vi "main_b.vi"(8 "error in (no error)":errorcluster, 10 "stages":refnum<class "_stage.lvclass">[](array[class]), 11 "_camera":refnum<class "_camera.lvclass">) -> ()   [LabVIEW 2019]
uses:
  _camera/_camera.lvlibp/_cameraClass/_camera.lvclass
  _stage/_stage.lvlibp/_stageClass/_stage.lvclass
  data_algorithm.ctl
  state.ctl
  data_process.ctl
  _data/_data.lvlibp/_dataClass/_data.lvclass
  <vilib>/Analysis/baseanly.llb/Mean (DBL).vi
  972fad81-3ff3-4c5b-b5d6-c93ea4aec52b.vi
  951adbdd-488d-47b0-b06c-8d69e9ccb4aa.vi
  2b97118a-447f-4295-80f1-8ed8751fa7ac.vi
  <vilib>/Utility/config.llb/Read Key (Path).vi
  <vilib>/Utility/config.llb/Read Key (String).vi
  _camera/_camera.lvlibp/_cameraClass/Write stage positions readback.vi
  _camera/_camera.lvlibp/_cameraClass/Write config file path.vi
  _camera/_camera.lvlibp/_cameraClass/Read camera name and version.vi
  _camera/_camera.lvlibp/_cameraClass/Write background.vi
  _camera/_camera.lvlibp/_cameraClass/Read wavelength.vi
  <vilib>/gmath/NumericalOptimization/Nonlinear Curve Fit LM formula string.vi
  _camera/_camera.lvlibp/_cameraClass/Write wavelength.vi
  _camera/_camera.lvlibp/_cameraClass/Read stage positions.vi
  _camera/_camera.lvlibp/_cameraClass/Write stage positions.vi
  <vilib>/Utility/file.llb/Read Delimited Spreadsheet (DBL).vi
  <vilib>/Utility/config.llb/Read Key (Double).vi
  <vilib>/Analysis/NI_AALBase.lvlib
  <vilib>/Utility/config.llb/NI_LVConfig.lvlib
  <vilib>/gmath/NI_Gmath.lvlib
  378a35e6-17c3-42fc-973f-4dbb75f37032.vi
  <vilib>/Utility/LVLibp/NI_PackedLibraryUtility.lvlib
panel:
  out "concatenated string":string
  out "t/out":bool
  in  "Tab Control 2":enum32{"Page 1", "Page 2"}(tab)
  out "number (0 to 1) 3":dbl
  in  "calibrate wavelength":bool caption="calibrate_wl"
  out "Boolean 3":bool
  out "number (0 to 1) 2":dbl
  out "number (0 to 1)":dbl
  out "size of dependent time scan":i32
  out "single acq. time":u32
  out "data proc. time":u32=150 caption="usec"
  in  "which plot":u16(ring)=2 items=["pumped", "unpumped", "reference", "difference"]
  in  "Algorithm":T1=3 items=["<(S*-S)/S>/ln(10)", "<S*/S>-1", "<S*/PD*>/<S/PD>", "<S*/Sref*>/<S/Sref>", "<S*/Sref*/PD*>/<S/Sref>", "<S*/Sref*>/<S/Sref>_alt"]
  in  "show reference spectrum?":bool
  in  "remove cursor":bool
  in  "add cursor":bool
  out "Array":i32[](array[numeric])
  out "x = y?":bool
  in  "reversed?":bool[](array[boolean])=[TRUE]
  in  "Experimenter":string="who are you?"
  in  "Title":string="A clever title"
  in  "Experimental parameters":string="sample:\nsolvent:\ncuvette:\noptical density:\nexcitation wavelength:\nexcitation power:\nexcitation spot size:\nexcitation fluence: \nprobe spot size:\ncomment:"
  out "current scan":i32
  in  "N scans":u16=5
  in  "sample":string="testSample"
  in  "Experiment":string="testExp"
  in  "center cursor":bool
  in  "save flag":bool
  in  "save type":bool[](array[boolean])=[FALSE, FALSE, FALSE, FALSE]
  in  "data folder":path=path "Z:/11 Setups/04 NOPA TA/01 Data"
  out "progress":dbl(slide)=21.0 scale=0.0..100.0
  out "scan progress":u8(slide)=16 scale=0.0..100.0
  out "Cursor position (wl)":dbl[](array[numeric]) format="%#.2g"
  out "Cursor position (idx)":dbl[](array[numeric])
  in  "ampl":cluster{dbl, dbl}(slide)={-0.2917505030181087, 6.9678068410462775} scale=-1.0..10.0
  in  "diff":dbl(slide)=26.28128772635815 scale=0.05..50.0
  out "main graph":cluster{"wavelength":dbl[], "ref mean":dbl[]}[](graph)
  out "Tab Control":T2(tab)
  out "Intensity Chart":dbl[][](graph)
  out "Intensity Graph":dbl[][](graph)
  out "Waveform Chart":T3(graph)
  out "std graph":cluster{"wavelength":dbl[], "ref std":dbl[]}[](graph)
  out "std":dbl
  out "std":dbl
  out "skipped":bool[](array[boolean])
  out "chopper out":bool[][](array[boolean])
  out "synchronization error":bool
  out "mean":dbl
  out "mean":dbl
  out "PD hist":T4(graph)
  out "PD":cluster{i32[], dbl[]}[](graph)
  in  "ts_plot_lin-log":bool caption="timestep_plot_linlog"
  out "base path":path
  out "stage config":path
  out "camera config":path
  out "Application Directory":path
  out "appended path":path
  out "Stage objects":refnum<class "_stage.lvclass">[](array[class])
  out "timesteps loaded from file":dbl[][](array[numeric])
  out "size of dependent time scan 2":i32
  out "Waveform Graph":dbl[](graph)
  in  "trig2 level":dbl(slide)=783.9195979899498 scale=0.0..2000.0
  out "Tank 2":dbl(slide) scale=0.0..2000.0
  out "Tank 2 + std":dbl(slide) scale=0.0..2000.0
  out "Tank 2 - std":dbl(slide) scale=0.0..2000.0
  in  "trig1 level":dbl(slide)=783.9195979899498 scale=0.0..2000.0
  out "Tank 1":dbl(slide)=552.7638190954774 scale=0.0..2000.0
  out "Tank 1 - std":dbl(slide) scale=0.0..2000.0
  out "Tank 1 + std":dbl(slide) scale=0.0..2000.0
  in  "baseline offset (ref.)":dbl
  in  "baseline offset (signal)":dbl
  in  "history length":i32=20
  in  "Scale.Range:Maximum":dbl(slide)=43.976036093027226 caption="diff scale range" scale=1.0..1000.0
  in  "camera max scale":u16(ring) items=["16-bit", "14-bit", "12-bit"]
  in  "save raw data":bool caption="saw raw data"
  in  "is measurement TA?":bool=TRUE
  out "Boolean 2":bool
  out "element 2":dbl
  out "element 3":dbl
  out "PDs mean":dbl[](array[numeric])
  out "PDs std":dbl[](array[numeric])
  out "dynamic offset":dbl[](array[numeric])
  in  "use dynamic offset?":bool
  in  "save wl calibration to .ini":bool caption="calibrate_wl"
  in  "index":u16
  out "wavelength fit":cluster{i32[], dbl[]}[](graph)
  out "wavelength (fitted)":dbl[](array[numeric]) format="%#.0f"
  in  "wavelength \n(calibration value)":dbl[](array[numeric]) caption="wavelength (calibration value)"
  in  "pixel/index":u16[](array[numeric])
  in  "mirror?":bool
  in  "initial parameters":dbl[](array[numeric])=[150.0, 200000.0, 1200.0]
  out "best fit parameters":dbl[](array[numeric])
  in  "time delay file":path=path "D:/github/TransientAbsorptionDAQ.lv/stepfiles/01_coarseSteps_-1000_1000fs.txt"
  in  "scan":bool
  in  "bottom panel":u16(ring)=2 items=["x/y", "y/x", "traces", "std", "debug", "debug 2", "parameters", "wavelength"]
  in  "parity?":enum32{"Item 0", "Item 1"}(radio)
  out "Camera initialised?":bool[](array[boolean])
  out "Char":i16
  in  "view error anal":bool
  in  "view full data":bool
  in  "get bg":bool
  in  "cont acq":bool
  in  "move stage":enum32{"Item 0", "Item 1"}(radio)
  out "timed out?":bool
  out "Boolean":bool
  out "Stage(s) initialized":bool[](array[boolean])
  in  "set as t0":bool[](array[boolean])
  in  "home stages":bool[](array[boolean])
  out "stage name(s)":i32[](listbox)
  in  "t0 position(s)":dbl[](array[numeric]) caption="t0 (s)" format="%07.0f"
  out "stage position(s) readback":dbl[](array[numeric]) caption="readback (fs)" format="%09.2f"
  in  "stage position(s)":dbl[](array[numeric]) caption="set (fs)" format="%07.0f"
  out "camera name, version":string
  in  "get_single_acq":bool caption="get single"
  out "vi running?":bool=TRUE
  out "is moving?":bool[](array[boolean]) caption="mov?"
  # "scan"
  # "out of"
  # "just temp ..."
  # "timing"
  # "usec"
  # "transient"
  # "pumped mean"
  # "unpumped mean"
  # "reference mean"
  # "Hartmann dispersion formula:"
  # "d(\\lambda) = a1 + a2 / (pix - a3)"
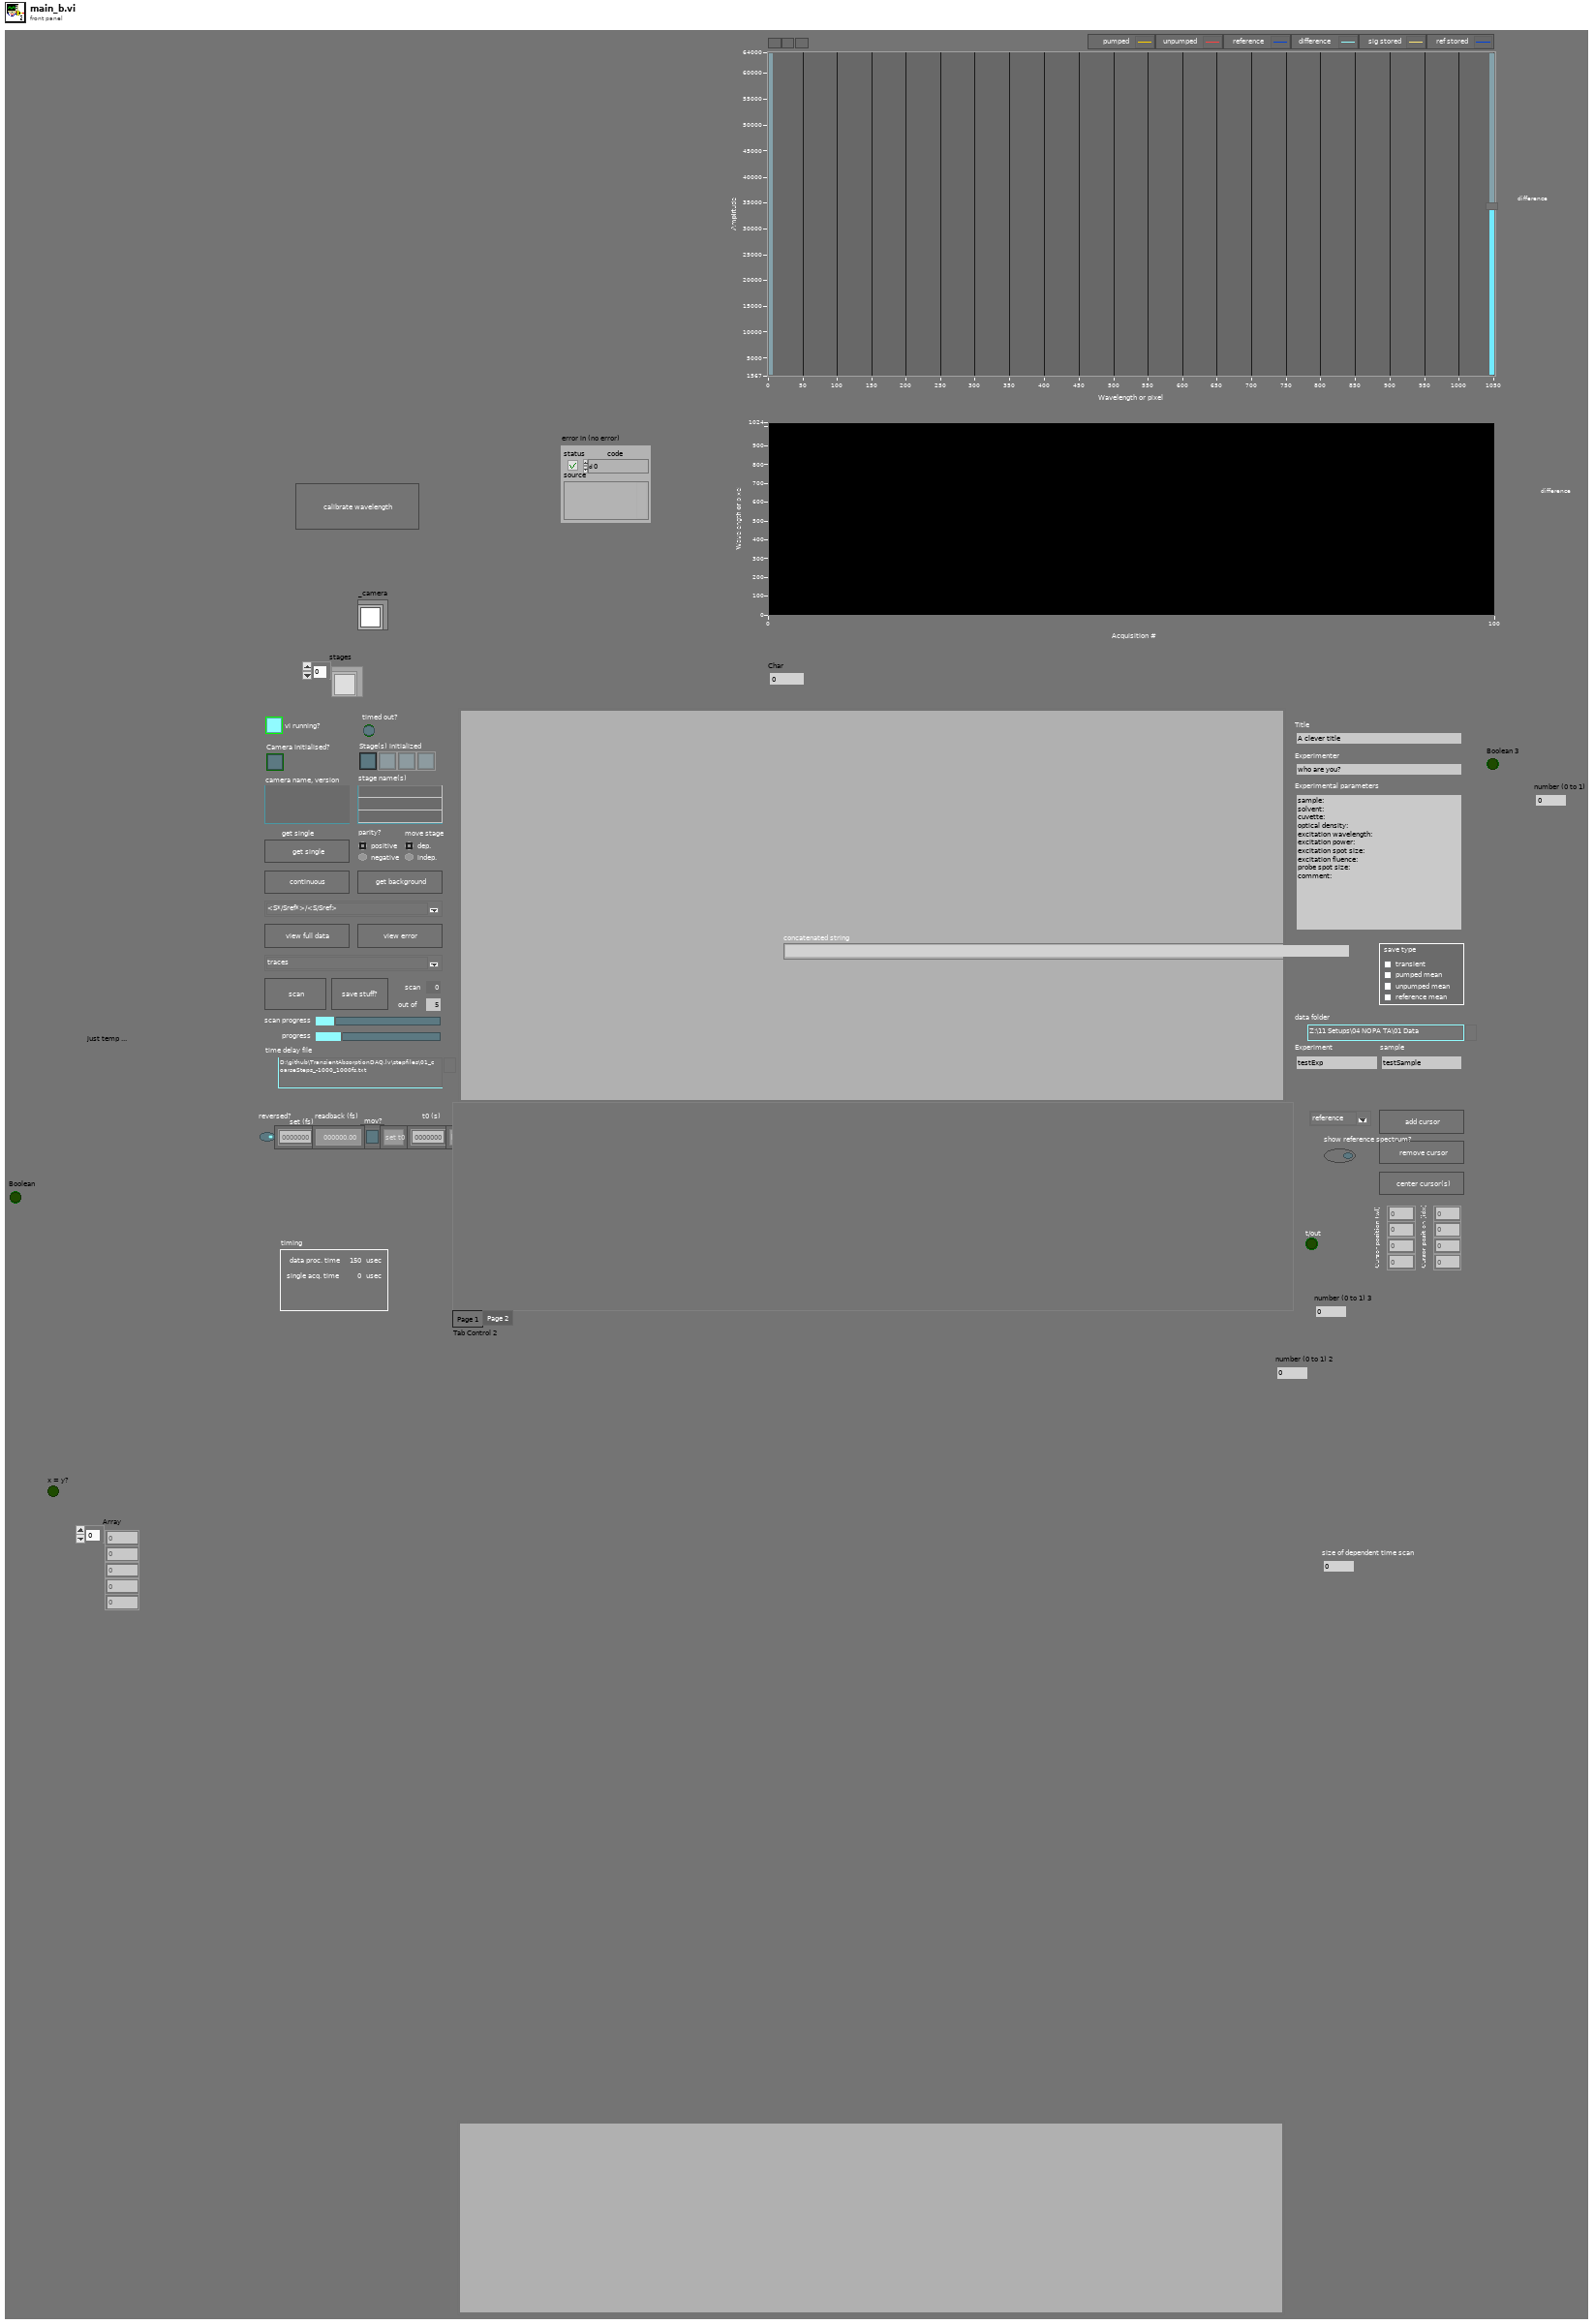
[diagram p1: front panel]
types:
  T1 = typedef "data_algorithm.ctl" = u16
  T2 = enum32{"x/y", "y/x", "traces", "std", "debug", "debug 2", "parameters", "wavelength"}
  T3 = cluster{"[0]":dbl, "[1]":dbl, "[2]":dbl, "[3]":dbl, "[4]":dbl, "[5]":dbl, "[6]":dbl, "[7]":dbl, "[8]":dbl}
  T4 = cluster{"Histogram: h(x)":i32[], "X Values":dbl[]}[]
  T5 = enum32{"invalid app kind", "Development System", "Run Time System", "Student Edition", "Embedded LabVIEW", "Evaluation", "Custom"}
  T6 = typedef "data_process.ctl" = enum16{"timeout", "init", "reset", "process", "plot", "save", "exit"}
  T7 = cluster{"type":string, "raw data":dbl[][][], "wavelength":dbl[], "trigger":bool[][], "stage position (set) [fs]":dbl[], "stage position (readback) [fs]":dbl[], "scn_step_pos (set)":dbl[], "scn_step_time_dly (set) [fs]":dbl[][], "scn_step":i32, "scn_iter":i32, "command":T6, "save flag":bool, "save path":path, "save type":bool[], "raw PDs":dbl[][]}
  T8 = typedef "state.ctl" = enum16{"timeout", "hw_init", "sw_init", "cam_single_acq", "cam_get_bg", "cam_rst_bg", "cam_cnt_acq", "cam_set_wl", "stg_set_pos", "stg_home", "scn_load_step_file", "scn_init", "scn_next_step", "scn_next_iter", "dat_update_save_flag", "dat_update_save_type", "dat_save_raw", "dat_send_to_process", "aux_save_wl_to_ini", "aux_center_cursor", "stop"}
  T9 = cluster{"acq num":u32[], "curr acq":i32, "signal":dbl[], "signal (accum.)":dbl[][], "pumped mean":dbl[], "unpumped mean":dbl[], "reference mean":dbl[], "pumped std":dbl[], "unpumped std":dbl[], "reference std":dbl[], "pumped stored":dbl[], "reference stored":dbl[], "signal std":dbl[]}
  T10 = typedef "NI_LVConfig.lvlib/Config Data RefNum.ctl" = refnum<k1>
  T11 = typedef "LVRangeTypeDef.ctl" = cluster{"Minimum":dbl, "Maximum":dbl, "Increment":dbl, "Minor Increment":dbl, "Start":dbl}
  T12 = typedef "LVCursorListTypeDef.ctl" = cluster{"Name":string, "Color":u32, "Style":u8, "Point Style":u8, "Name Visible":bool, "Allow Drag":bool, "Cursor Mode":u32, "Plot":i32, "Index":i32, "Position":cluster{"X":dbl, "Y":dbl}, "X Scale":u32, "Y Scale":u32, "Watch Plots":i32[], "Watch All Plots":bool, "Plot Area":i32, "Label Offset":cluster{"X":dbl, "Y":dbl}}[]
  T13 = cluster{"Name":string, "Color":u32, "Style":u8, "Point Style":u8, "Name Visible":bool, "Allow Drag":bool, "Cursor Mode":u32, "Plot":i32, "Index":i32, "Position":cluster{"X":dbl, "Y":dbl}, "X Scale":u32, "Y Scale":u32, "Watch Plots":i32[], "Watch All Plots":bool, "Plot Area":i32, "Label Offset":cluster{"X":dbl, "Y":dbl}}
  T14 = cluster{"wavelength":dbl[], "unpumped mean":dbl[]}
  T15 = cluster{"wavelength":dbl[], "reference mean":dbl[]}
  T16 = cluster{"wavelength":dbl[], "reference stored":dbl[]}
  T17 = cluster{"wavelength":dbl[], "pumped stored":dbl[]}
  T18 = cluster{"Histogram: h(x)":i32[], "X Values":dbl[]}
  T19 = cluster{"wavelength":dbl[], "reference stored":dbl[]}[]
  T20 = cluster{"wavelength":dbl[], "unpumped std":dbl[]}
  T21 = cluster{"wavelength":dbl[], "reference std":dbl[]}
  T22 = cluster{"wavelength":dbl[], "reference std":dbl[]}[]
  T23 = cluster{"model":string, "Parameters":string[], "x":string}
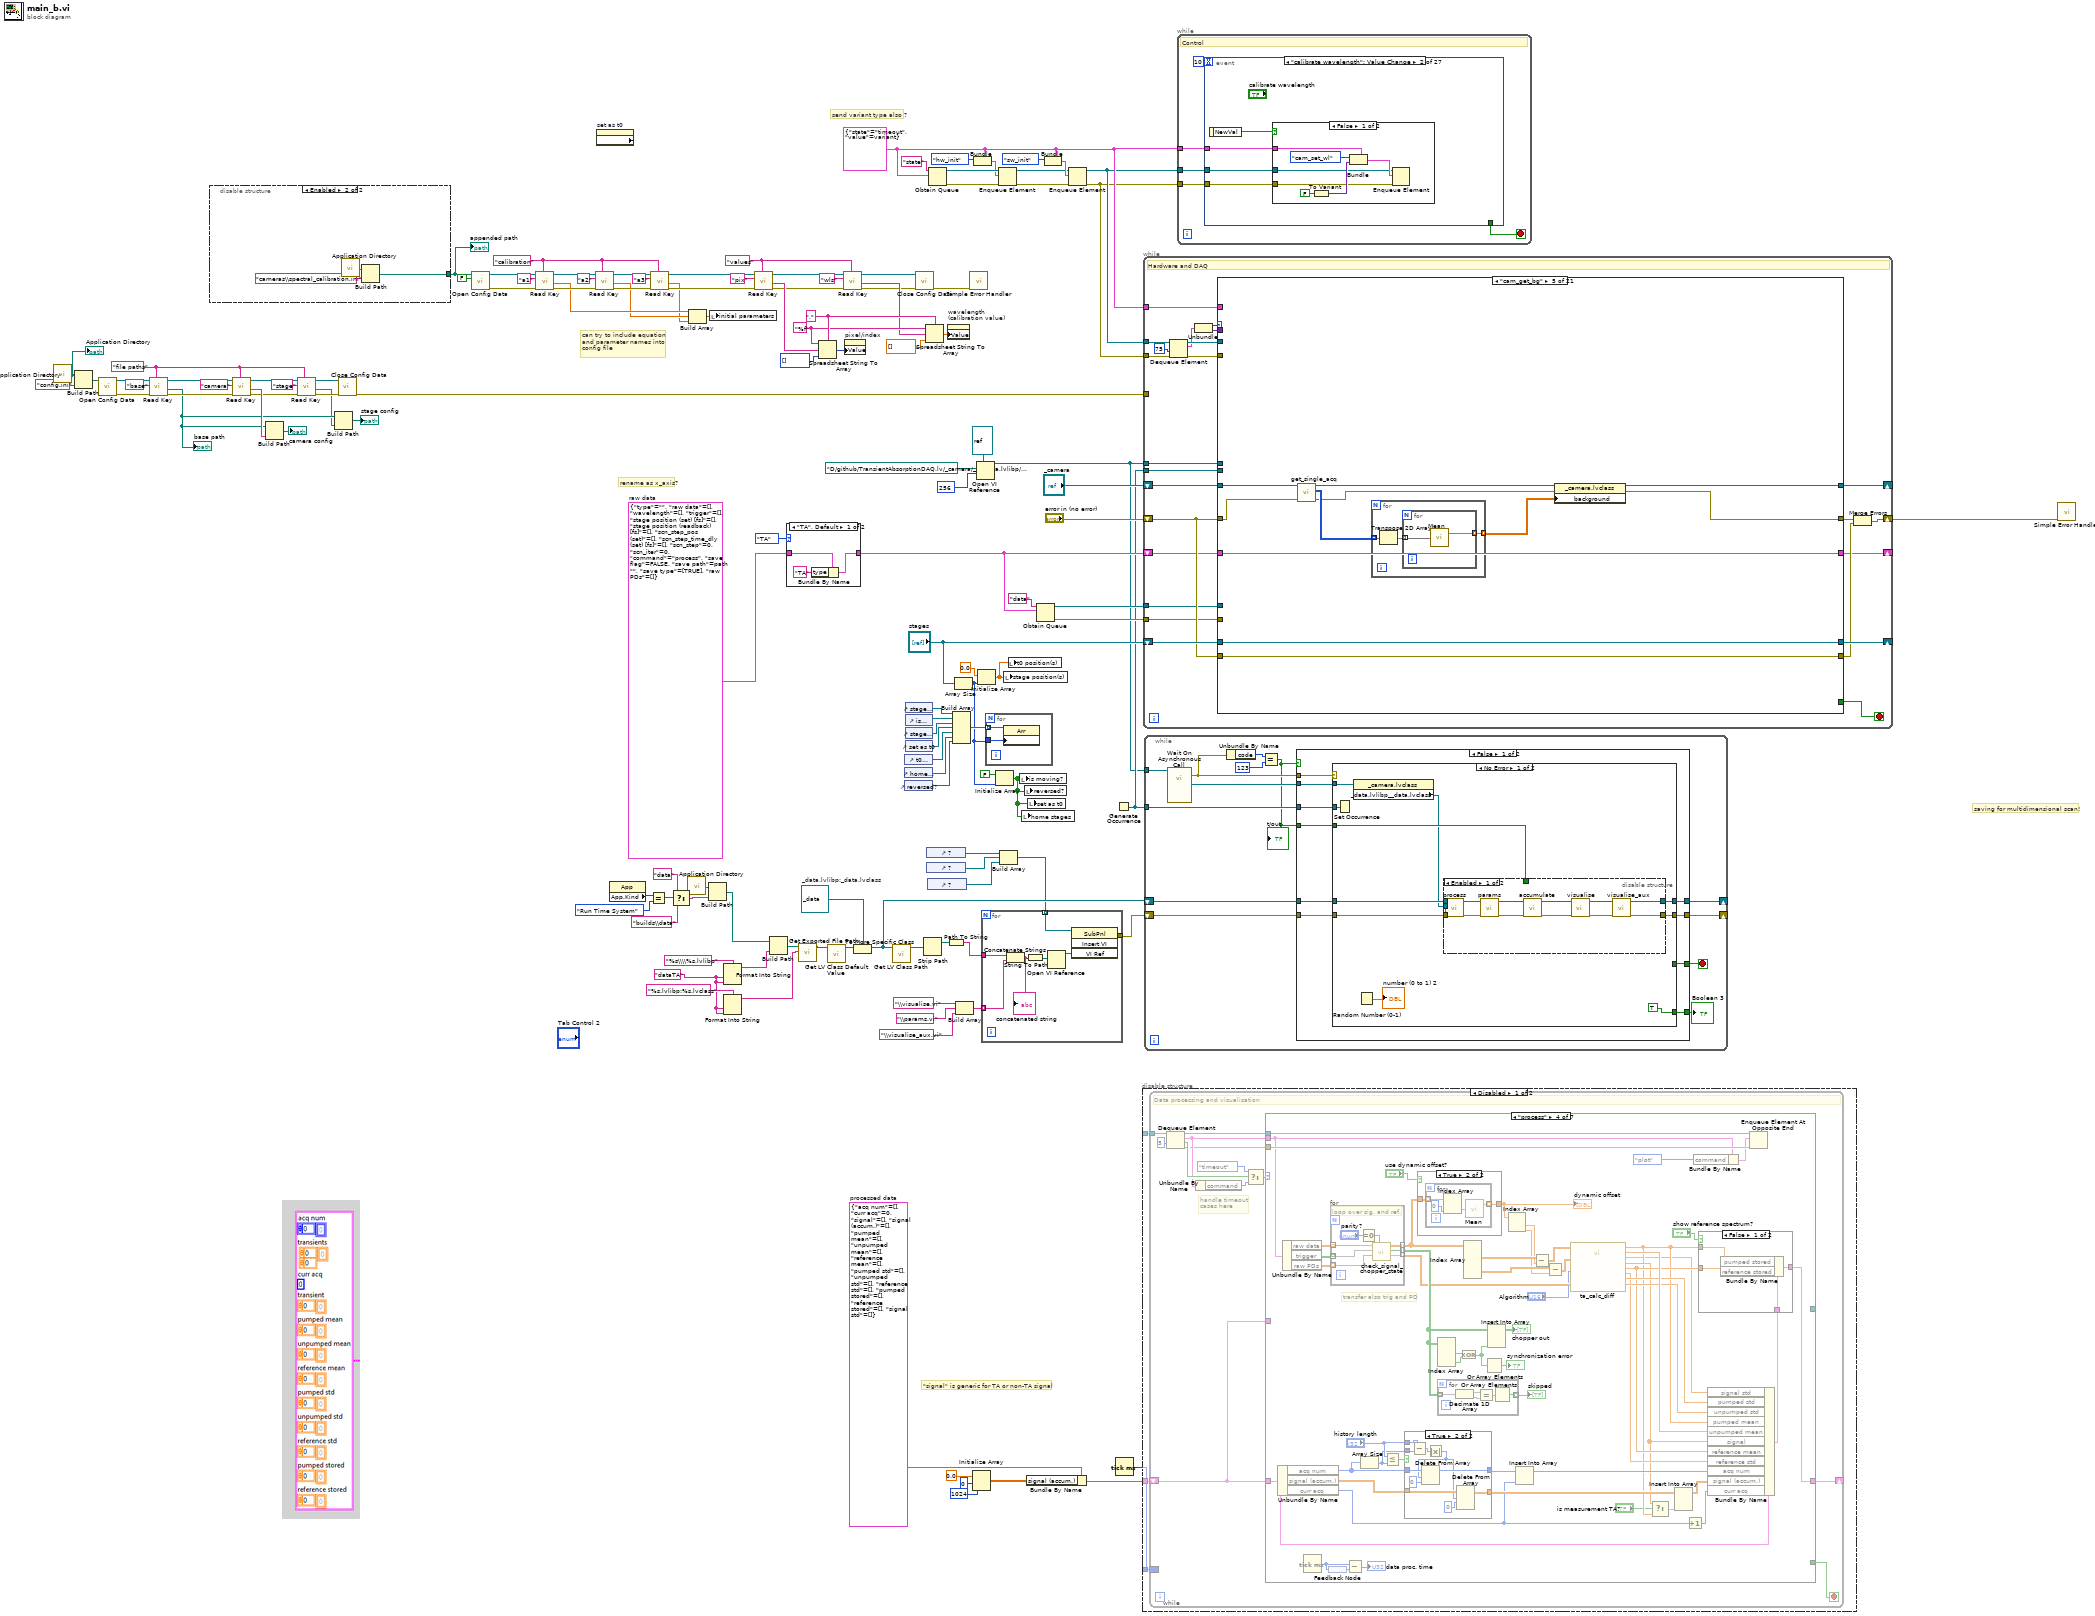
[diagram p0: block diagram]
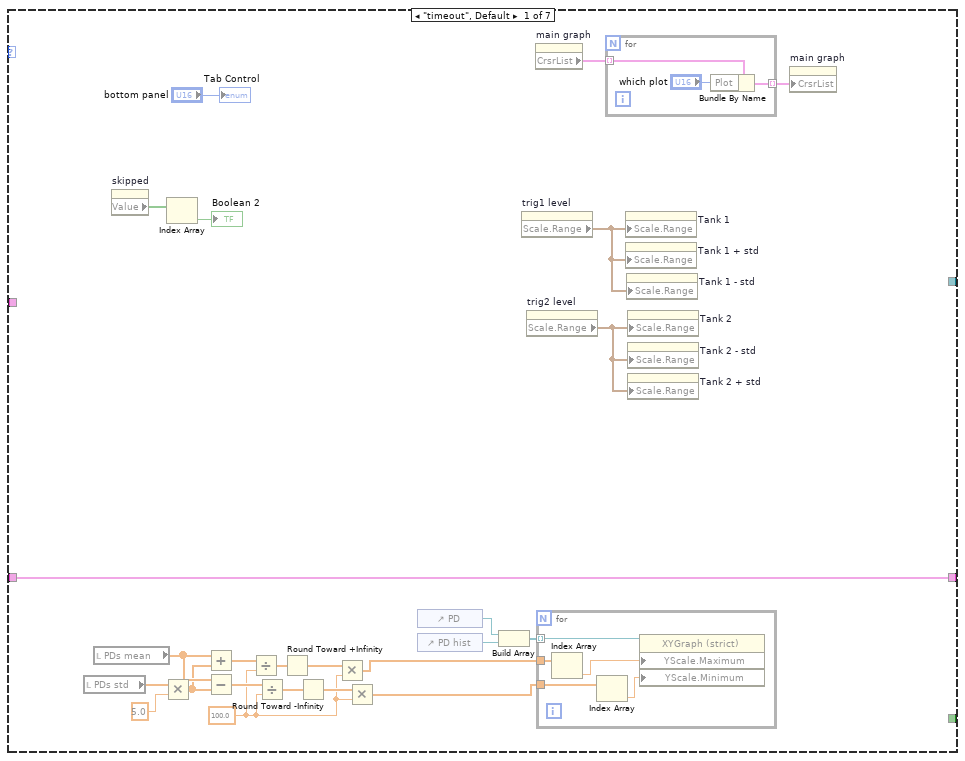
[diagram p2: hidden frame]
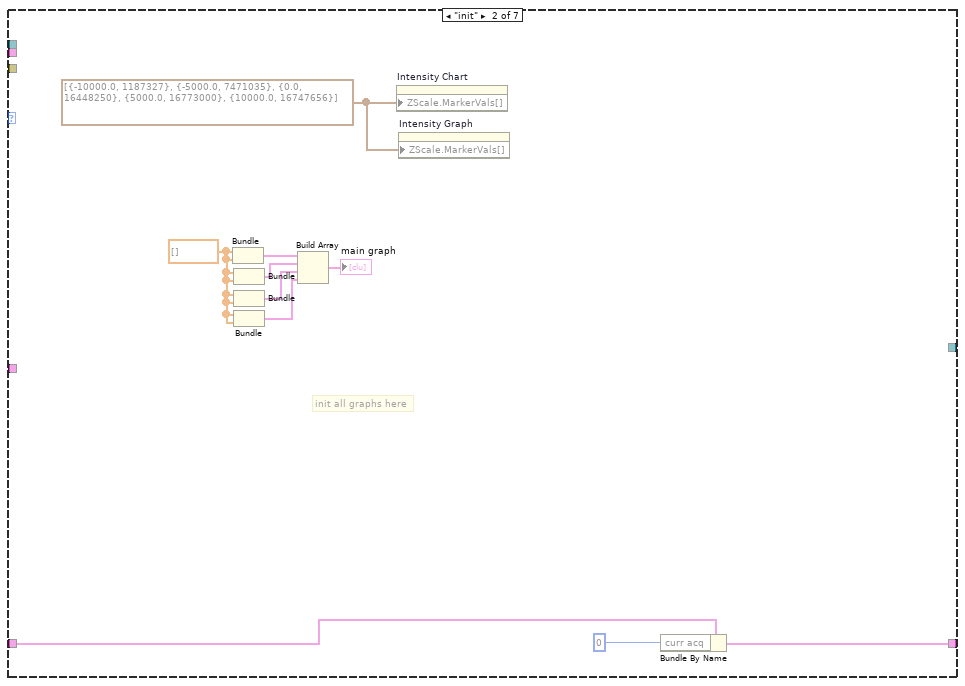
[diagram p3: hidden frame]
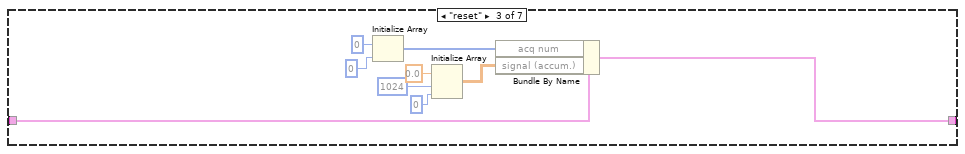
[diagram p4: hidden frame]
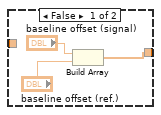
[diagram p5: hidden frame]
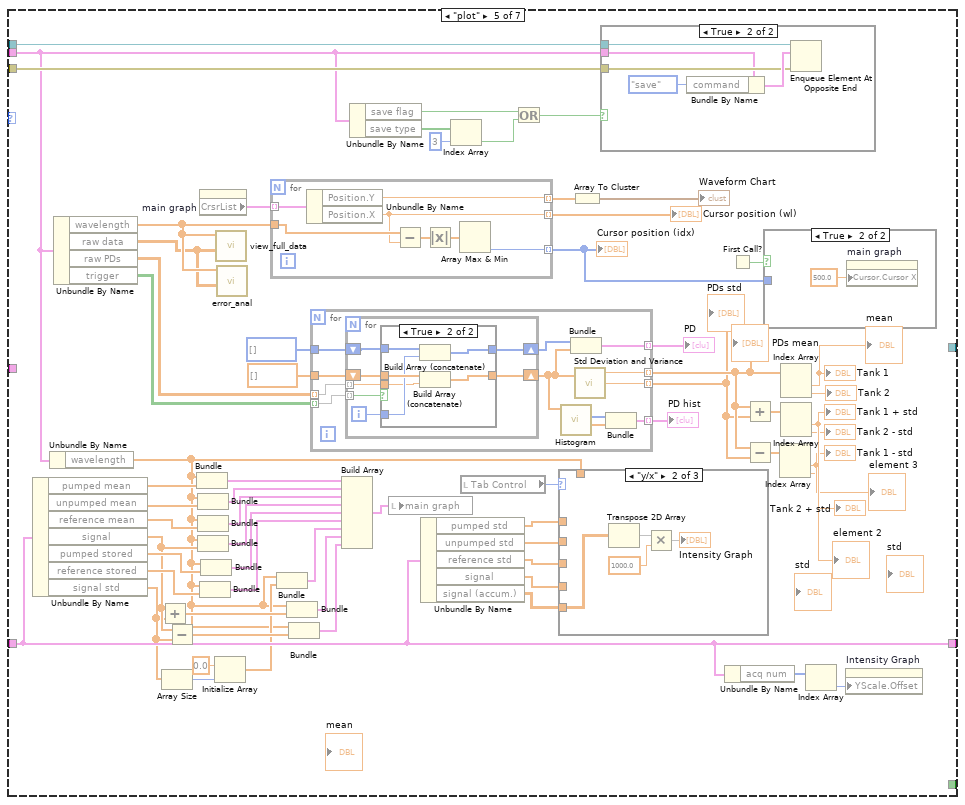
[diagram p8: hidden frame]
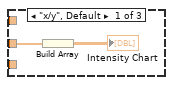
[diagram p12: hidden frame]
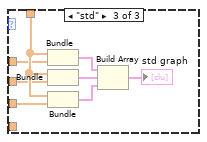
[diagram p13: hidden frame]
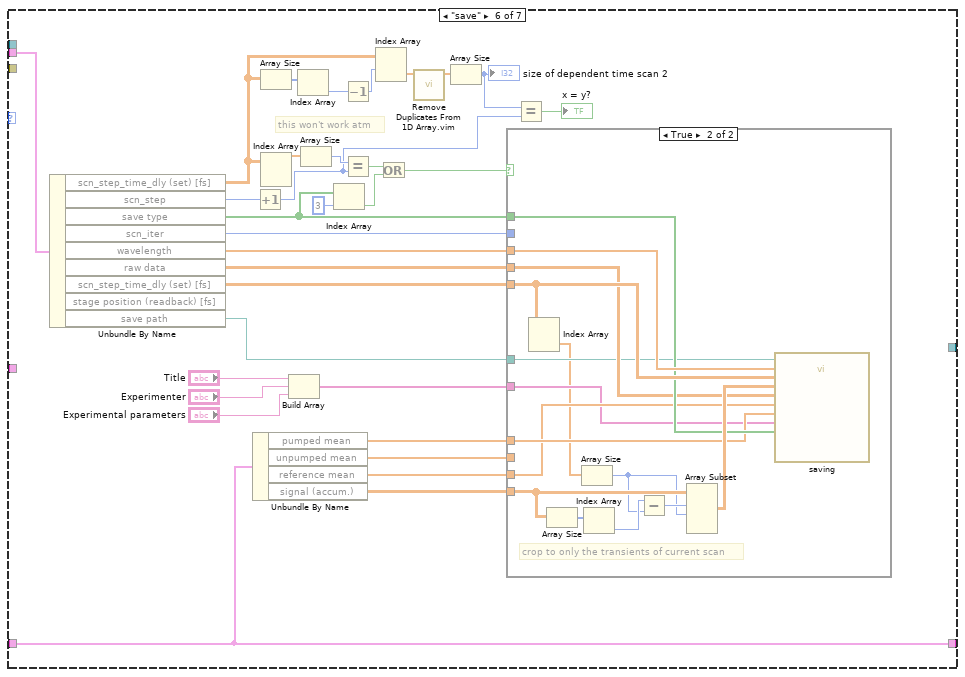
[diagram p14: hidden frame]
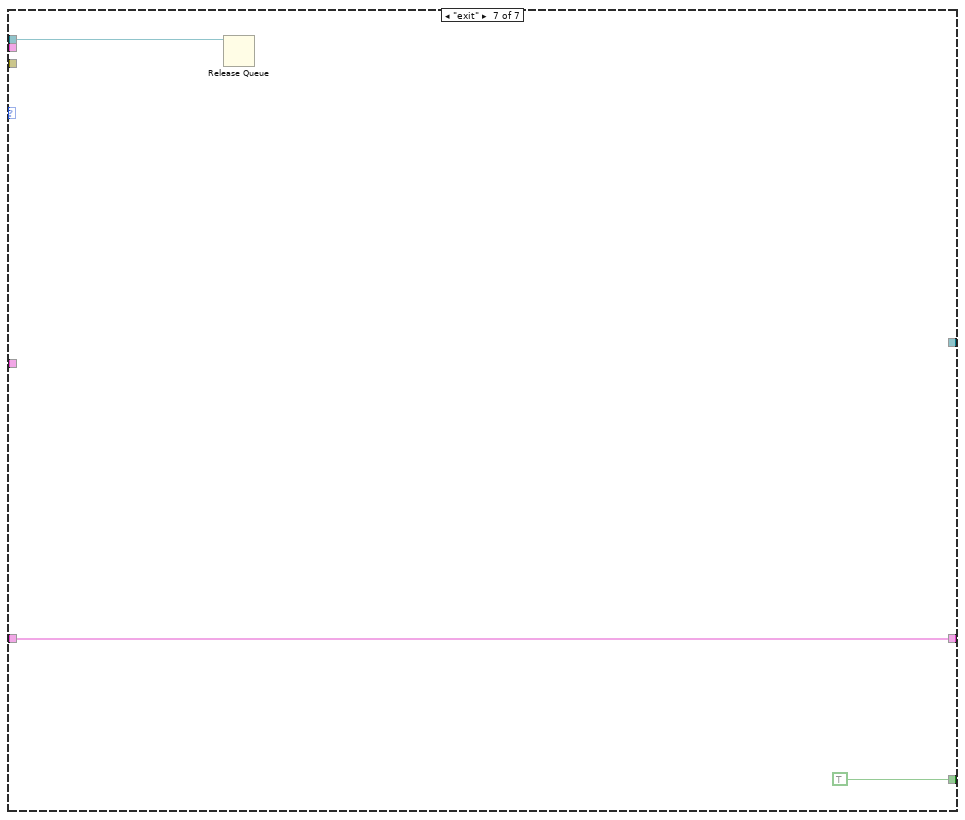
[diagram p16: hidden frame]
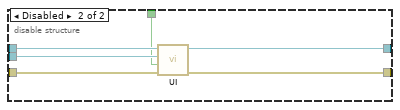
[diagram p18: hidden frame]
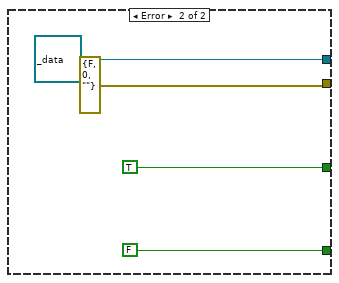
[diagram p19: hidden frame]
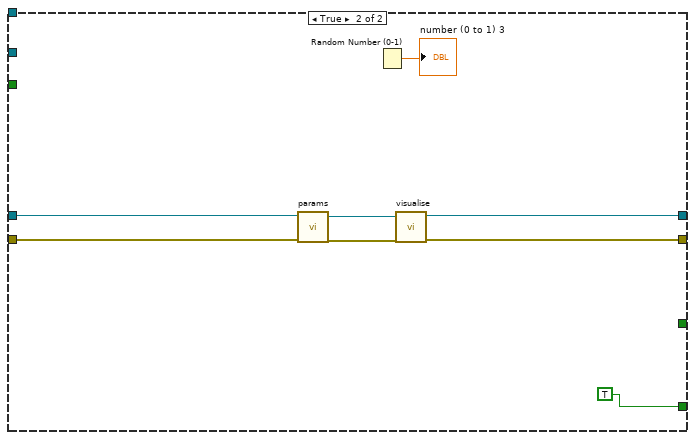
[diagram p20: hidden frame]
diagram:
  w18 = "dataTA"
  w35 = refnum<class "_data.lvclass"> refnum  # _data.lvlibp:_data.lvclass
  w38 = T7 {"type"="", "raw data"=[], "wavelength"=[], "trigger"=[], "stage position (set) [fs]"=[], "stage position (readback) [fs]"=[], "scn_step_pos (set)"=[], "scn_step_time_dly (set) [fs]"=[], "scn_step"=0, "scn_iter"=0, "command"=enum."process", "save flag"=FALSE, "save path"=path "", "save type"=[TRUE], "raw PDs"=[]}  # raw data
  w42 = "file paths" ("section")
  w80 = "," ("delimiter (Tab)")
  w79 = "%f" ("format string")
  w81 = "values" ("section")
  w95 = "calibration" ("section")
  w37 = T9 {"acq num"=[], "curr acq"=0, "signal"=[], "signal (accum.)"=[], "pumped mean"=[], "unpumped mean"=[], "reference mean"=[], "pumped std"=[], "unpumped std"=[], "reference std"=[], "pumped stored"=[], "reference stored"=[], "signal std"=[]}  # processed data
  w69 = cluster{"state":T8, "value":variant} {"state"=enum."timeout", "value"=variant}
  # "saving for multidimensional scan!"
  # "\"signal\" is generic for TA or non-TA signal"
  # "rename as x_axis?"
  # "can try to include equation\nand parameter names into \nconfig file"
  # "send variant type also ?"
  n1 = call <vilib>:"Application Directory.vi"() -> ("Application Directory"=w57:path)
  "Application Directory" <- w57
  n2 = Build Path(base path=w57, name or relative path="config.ini") -> (appended path=w55:path)
  n3 = call <vilib>:"Open Config Data.vi"("configuration file path"=w55) -> ("error out"=w59:errorcluster, "refnum"=w60:T10)  [unwired: 8 in, 1 out]
  n4 = call-poly <vilib>:"Read Key.vi"("section"=w42, "error in (no error)"=w59, "key"="base", "refnum"=w60) -> ("error out"=w49:errorcluster, "value"=w47:path, "refnum out"=w50:T10)  [unwired: 4 in, 1 out]
  "base path" <- w47
  n5 = disable-structure shown="Enabled" {
    disable-tunnel: [w143 w144] -> w101
    frame Disabled {
      n6 = property class="App"() -> ("App.Kind"=w140:T5)  [unwired: 2 in, 2 out]
      n7 = Equal?(x=w140, y=T5."Run Time System") -> (x = y?=w138:bool)
      n8 = Select(t="cameras" ("name or relative path"), s=w138, f="builds\\cameras" ("name or relative path")) -> (s? t:f=w135:string)
      n9 = call <vilib>:"Application Directory.vi"() -> ("Application Directory"=w142:path)
      n10 = Build Path(base path=w142, name or relative path=w135) -> (appended path=w141:path)
      n11 = call "File Dialog"("start path"=w141, "prompt"="select spectral calibration", "pattern (all files)"="*.ini") -> ("selected path"=w143:path)  [unwired: 9 in, 3 out]
    }
    frame Enabled {
      n12 = call <vilib>:"Application Directory.vi"() -> ("Application Directory"=w146:path)
      n13 = Build Path(base path=w146, name or relative path="cameras\\spectral_calibration.ini") -> (appended path=w144:path)
    }
  }
  "appended path" <- w101
  n14 = call-poly <vilib>:"Read Key.vi"("section"=w42, "error in (no error)"=w49, "key"="camera", "refnum"=w50) -> ("error out"=w44:errorcluster, "value"=w48:string, "refnum out"=w43:T10)  [unwired: 4 in, 1 out]
  n15 = Build Path(base path=w47, name or relative path=w48) -> (appended path=→"camera config":path)
  n16 = call-poly <vilib>:"Read Key.vi"("section"=w42, "error in (no error)"=w44, "key"="stage", "refnum"=w43) -> ("error out"=w52:errorcluster, "value"=w46:string, "refnum out"=w53:T10)  [unwired: 4 in, 1 out]
  n17 = Build Path(base path=w47, name or relative path=w46) -> (appended path=→"stage config":path)
  n18 = call <vilib>:"Close Config Data.vi"("error in (no error)"=w52, "refnum"=w53) -> ("error out"=w40:errorcluster)  [unwired: 8 in, 1 out]
  n19 = call <vilib>:"Open Config Data.vi"("create file if necessary (T)"=FALSE, "configuration file path"=w101) -> ("error out"=w99:errorcluster, "refnum"=w100:T10)  [unwired: 7 in, 1 out]
  n20 = call-poly <vilib>:"Read Key.vi"("section"=w95, "error in (no error)"=w99, "key"="a1", "refnum"=w100) -> ("error out"=w93:errorcluster, "value"=w64:dbl, "refnum out"=w94:T10)  [unwired: 4 in, 1 out]
  n21 = call-poly <vilib>:"Read Key.vi"("section"=w95, "error in (no error)"=w93, "key"="a2", "refnum"=w94) -> ("error out"=w92:errorcluster, "value"=w63:dbl, "refnum out"=w91:T10)  [unwired: 4 in, 1 out]
  n22 = property on="set as t0" class="Arr" props=["Number of Rows"]() -> ()  [unwired: 2 in, 3 out]
  n23 = property class="App"() -> ("App.Kind"=w30:T5)  [unwired: 2 in, 2 out]
  n24 = Equal?(x=w30, y=T5."Run Time System") -> (x = y?=w28:bool)
  n25 = call-poly <vilib>:"Read Key.vi"("section"=w95, "error in (no error)"=w92, "key"="a3", "refnum"=w91) -> ("error out"=w89:errorcluster, "value"=w62:dbl, "refnum out"=w90:T10)  [unwired: 4 in, 1 out]
  n26 = Select(t="data" ("name or relative path"), s=w28, f="builds\\data" ("name or relative path")) -> (s? t:f=w25:string)
  n27 = call <vilib>:"Application Directory.vi"() -> ("Application Directory"=w31:path)
  n28 = Build Array(w64, w63, w62) -> (w61:dbl[])
  n29 = Build Path(base path=w31, name or relative path=w25) -> (appended path=w19:path)
  n30 = local write "initial parameters"(w61) -> ()
  n31 = Format Into String(format string="%s\\\\%s.lvlibp", w18, w18) -> (resulting string=w22:string)  [unwired: 2 in, 1 out]
  n32 = Format Into String(format string="%s.lvlibp:%s.lvclass", w18, w18) -> (resulting string=w23:string)  [unwired: 2 in, 1 out]
  n33 = call-poly <vilib>:"Read Key.vi"("section"=w81, "error in (no error)"=w89, "key"="pix", "refnum"=w90) -> ("error out"=w82:errorcluster, "value"=w88:string, "refnum out"=w83:T10)  [unwired: 4 in, 1 out]
  n34 = Build Path(base path=w19, name or relative path=w22) -> (appended path=w24:path)
  n35 = case shown="\"TA\", Default" enum16{"TA", "2D"}."TA" {
    tunnel: [w147 w151] -> w104
    tunnel: w38 -> [w149 w152]
    frame "TA", Default {
      n36 = Bundle By Name(cluster=w149, "type"="TA") -> (w147:T7)
    }
    frame "2D" {
      n37 = Bundle By Name(cluster=w152, "type"="2D") -> (w151:T7)
    }
  }
  n38 = call <vilib>:"Get Exported File Path.vi"("qualified name"=w23, "packed library path"=w24) -> ("path"=w17:path)  [unwired: 8 in, 1 out]
  n39 = Spreadsheet String To Array(delimiter (Tab)=w80, format string=w79, spreadsheet string=w88, array type (2D Dbl)=i32[] []) -> (array=w85:i32[])
  n40 = call <vilib>:"Get LV Class Default Value.vi"("class path"=w17) -> ("object"=w36:refnum<class>)  [unwired: 9 in, 1 out]
  n41 = call-poly <vilib>:"Read Key.vi"("section"=w81, "error in (no error)"=w82, "key"="wls", "refnum"=w83) -> ("error out"=w74:errorcluster, "value"=w78:string, "refnum out"=w75:T10)  [unwired: 4 in, 1 out]
  n42 = property on="pixel/index" class="Arr (strict)"("Value"=w85) -> ()  [unwired: 2 in, 2 out]
  n43 = To More Specific Class(target class=w35, reference=w36) -> (specific class reference=w34:refnum<class "_data.lvclass">)  [unwired: 1 in, 1 out]
  n44 = call <vilib>:"Get LV Class Path.vi"("object"=w34) -> ("class path"=w10:path)  [unwired: 9 in, 1 out]
  n45 = control-ref of="t0 position(s)"() -> (w118:refnum<vi>)
  n46 = control-ref of="home stages"() -> (w117:refnum<vi>)
  n47 = control-ref of="reversed?"() -> (w66:refnum<vi>)
  n48 = control-ref of="stage position(s)"() -> (w120:refnum<vi>)
  n49 = control-ref of="is moving?"() -> (w123:refnum<vi>)
  n50 = control-ref of="stage position(s) readback"() -> (w122:refnum<vi>)
  n51 = control-ref of="set as t0"() -> (w119:refnum<vi>)
  n52 = call <vilib>:"Close Config Data.vi"("error in (no error)"=w74, "refnum"=w75) -> ("error out"=w9:errorcluster)  [unwired: 8 in, 1 out]
  n53 = Strip Path(path=w10) -> (stripped path=w32:path)  [unwired: 1 out]
  n54 = Spreadsheet String To Array(delimiter (Tab)=w80, format string=w79, spreadsheet string=w78, array type (2D Dbl)=dbl[] []) -> (array=w76:dbl[])
  n55 = control-ref of="?"() -> (w8:refnum<vi>)
  n56 = control-ref of="?"() -> (w7:refnum<vi>)
  n57 = control-ref of="?"() -> (w6:refnum<vi>)
  n58 = Obtain Queue(name (unnamed)="state", element data type=w69) -> (queue out=w130:refnum<queue>, error out=w129:errorcluster)  [unwired: 3 in, 1 out]
  n59 = Path To String(path=w32) -> (string=w33:string)
  n60 = property on="wavelength \n(calibration value)" class="Arr (strict)"("Value"=w76) -> ()  [unwired: 2 in, 2 out]
  n61 = Build Array(w120, w123, w122, w119, w118, w117, w66) -> (w121:refnum<vi>[])
  n62 = Array Size(array="stages") -> (size(s)=w114:i32)
  n63 = Build Array("\\visualise.vi" ("string"), "\\params.vi" ("string"), "\\visualise_aux.vi" ("string")) -> (w1:string[])
  n64 = call <vilib>:"Simple Error Handler.vi"("error in (no error)"=w9) -> ()  [unwired: 4 in, 5 out]
  n65 = Initialize Array(0.0, 0 ("dimension size"), 1024 ("dimension size")) -> (w108:dbl[][])
  n66 = Bundle(cluster=w69, "state"=state."hw_init") -> (w116:cluster{"state":T8, "value":variant})  [unwired: 1 in]
  n67 = Open VI Reference(type specifier VI Refnum (for type only)=refnum<vi> refnum, vi path=path "D:/github/TransientAbsorptionDAQ.lv/_camera/_camera.lvlibp/_cameraClass/get_single_acq_wrapper.vi", options=256) -> (vi reference=w12:refnum<vi>)  [unwired: 3 in, 1 out]
  n68 = Initialize Array(0.0, w114) -> (w113:dbl[])
  n69 = for {
    tunnel: w121 -> [w153] mode=indexing
    tunnel: w114 -> [w154]
    n70 = property class="Arr"(reference=w153, "Number of Rows"=w154) -> ()  [unwired: 1 in, 2 out]
  }
  n71 = Initialize Array(FALSE, w114) -> (w65:bool[])
  n72 = Enqueue Element(queue=w130, element=w116, error in (no error)=w129) -> (queue out=w71:refnum<queue>, error out=w70:errorcluster)  [unwired: 1 in, 1 out]
  n73 = Build Array(w8, w7, w6) -> (w2:refnum<vi>[])
  n74 = for {
    tunnel: w33 -> [w160]
    tunnel: [w157] -> w11
    tunnel: w2 -> [w156] mode=indexing
    tunnel: w1 -> [w155] mode=indexing
    n75 = Concatenate Strings(w160, w155) -> (w159:string)
    "concatenated string" <- w159
    n76 = String To Path(string=w159) -> (path=w158:path)
    n77 = Open VI Reference(vi path=w158) -> (vi reference=w161:refnum<vi>)  [unwired: 5 in, 1 out]
    n78 = invoke class="SubPnl" method="Insert VI"(reference=w156, "VI Ref"=w161) -> (error out=w157:errorcluster)  [unwired: 2 in, 3 out]
  }
  n79 = local write "stage position(s)"(w113) -> ()
  n80 = local write "t0 position(s)"(w113) -> ()
  n81 = local write "is moving?"(w65) -> ()
  n82 = local write "home stages"(w65) -> ()
  n83 = local write "reversed?"(w65) -> ()
  n84 = Bundle By Name(cluster=w37, "signal (accum.)"=w108) -> (w109:T9)
  n85 = local write "set as t0"(w65) -> ()
  n86 = Obtain Queue(name (unnamed)="data", element data type=w104) -> (queue out=w103:refnum<queue>, error out=w105:errorcluster)  [unwired: 3 in, 1 out]
  n87 = Bundle(cluster=w69, "state"=state."sw_init") -> (w73:cluster{"state":T8, "value":variant})  [unwired: 1 in]
  n88 = Enqueue Element(queue=w71, element=w73, error in (no error)=w70) -> (queue out=w68:refnum<queue>, error out=w67:errorcluster)  [unwired: 1 in, 1 out]
  n89 = Generate Occurrence() -> (w13:refnum<k4>)
  n90 = Tick Count (ms)() -> (millisecond timer value=w124:u32)
  n91 = disable-structure shown="Disabled" {
    disable-tunnel: w124 -> [w164 _]
    disable-tunnel: w109 -> [w163 _]
    disable-tunnel: _ -> [w162 _]
    frame Disabled {
      n92 = while {
        border: w164 -> [_]
        shift-right: [w165] -> _
        shift-left: w163 -> [w166]
        tunnel: w162 -> [w173]
        stop <- w176 stop-if-true
        # "handle timeout\ncases here"
        # "Data processing and visualisation"
        n93 = Dequeue Element(queue=w173, timeout in ms (-1)=5) -> (queue out=w170:refnum<queue>, element=w169:T7, timed out?=w171:bool, error out=w168:errorcluster)  [unwired: 1 in]
        n94 = Unbundle By Name(w169) -> ("command"=w167:T6)
        n95 = Select(t=data_process."timeout", s=w171, f=w167) -> (s? t:f=w174:T6)
        n96 = case shown="\"process\"" w174 {
          tunnel: [_ _ _ _ _ _ TRUE] -> w176
          tunnel: w166 -> [w200 w217 w222 w264 w372 w469 w488]
          tunnel: [w200 w215 w219 w247 w372 w469 w488] -> w165
          tunnel: w170 -> [_ _ _ w261 w365 _ w487]
          tunnel: w169 -> [_ _ _ w228 w363 w471 _]
          tunnel: w168 -> [_ _ _ w260 w364 _ _]
          tunnel: _ -> [_ _ _ _ w321 _ _]
          tunnel: w166 -> [_ _ _ _ _ _ _]
          frame "timeout", Default {
            w179 = 100.0
            n97 = local read "PDs std"() -> (w191:dbl[])
            n98 = local read "PDs mean"() -> (w192:dbl[])
            n99 = property on="skipped" class="Arr (strict)"() -> ("Value"=w196:bool[])  [unwired: 2 in, 2 out]
            n100 = Multiply(x=w191, y=5.0) -> (x*y=w190:dbl[])
            n101 = Index Array(array=w196) -> (element=→"Boolean 2":bool)  [unwired: 1 in]
            n102 = Add(x=w192, y=w190) -> (x+y=w185:dbl[])
            n103 = Subtract(x=w192, y=w190) -> (x-y=w184:dbl[])
            n104 = Divide(x=w185, y=w179) -> (x/y=w183:dbl[])
            n105 = Divide(x=w184, y=w179) -> (x/y=w182:dbl[])
            n106 = Round Toward +Infinity(x=w183) -> (ceil(x): smallest int >= x=w181:dbl[])
            n107 = Round Toward -Infinity(1:w182) -> (0:w180:dbl[])
            n108 = Multiply(x=w181, y=w179) -> (x*y=w178:dbl[])
            n109 = Multiply(x=w180, y=w179) -> (x*y=w177:dbl[])
            n110 = control-ref of="PD"() -> (w188:refnum<vi>)
            n111 = control-ref of="PD hist"() -> (w187:refnum<vi>)
            n112 = Build Array(w188, w187) -> (w186:refnum<vi>[])
            n113 = property on="trig1 level" class="Slide (strict)"() -> ("Scale.Range"=w194:T11)  [unwired: 2 in, 2 out]
            n114 = property on="trig2 level" class="Slide (strict)"() -> ("Scale.Range"=w193:T11)  [unwired: 2 in, 2 out]
            n115 = property on="main graph" class="XYGraph (strict)"() -> ("CrsrList"=w197:T12)  [unwired: 2 in, 2 out]
            n116 = for {
              tunnel: w186 -> [w205] mode=indexing
              tunnel: w178 -> [w204]
              tunnel: w177 -> [w202]
              n117 = Index Array(array=w204) -> (element=w203:dbl)  [unwired: 1 in]
              n118 = Index Array(array=w202) -> (element=w201:dbl)  [unwired: 1 in]
              n119 = property on="Property Node" class="XYGraph (strict)"(reference=w205, "YScale.Maximum"=w203, "YScale.Minimum"=w201) -> ()  [unwired: 1 in, 2 out]
            }
            n120 = for {
              tunnel: [w208] -> w198 mode=indexing
              tunnel: w197 -> [w207] mode=indexing
              n121 = Bundle By Name(cluster=w207, "Plot"="which plot") -> (w208:T13)
            }
            n122 = property on="Tank 1" class="Slide (strict)"("Scale.Range"=w194) -> ()  [unwired: 2 in, 2 out]
            n123 = property on="Tank 1 + std" class="Slide (strict)"("Scale.Range"=w194) -> ()  [unwired: 2 in, 2 out]
            n124 = property on="Tank 1 - std" class="Slide (strict)"("Scale.Range"=w194) -> ()  [unwired: 2 in, 2 out]
            n125 = property on="Tank 2" class="Slide (strict)"("Scale.Range"=w193) -> ()  [unwired: 2 in, 2 out]
            n126 = property on="Tank 2 - std" class="Slide (strict)"("Scale.Range"=w193) -> ()  [unwired: 2 in, 2 out]
            n127 = property on="Tank 2 + std" class="Slide (strict)"("Scale.Range"=w193) -> ()  [unwired: 2 in, 2 out]
            n128 = property on="main graph" class="XYGraph (strict)"("CrsrList"=w198) -> ()  [unwired: 2 in, 2 out]
            "Tab Control" <- "bottom panel"
          }
          frame "init" {
            w209 = dbl[] []
            w218 = cluster{dbl, u32}[] [{-10000.0, 1187327}, {-5000.0, 7471035}, {0.0, 16448250}, {5000.0, 16773000}, {10000.0, 16747656}] ("Z Scale.Marker Values[]")
            # "init all graphs here"
            n129 = Bundle(w209, w209) -> (w214:cluster{dbl[], dbl[]})  [unwired: 1 in]
            n130 = Bundle(w209, w209) -> (w213:cluster{dbl[], dbl[]})  [unwired: 1 in]
            n131 = Bundle(w209, w209) -> (w212:cluster{dbl[], dbl[]})  [unwired: 1 in]
            n132 = Bundle(w209, w209) -> (w211:cluster{dbl[], dbl[]})  [unwired: 1 in]
            n133 = Build Array(w214, w213, w212, w211) -> (→"main graph":cluster{dbl[], dbl[]}[])
            n134 = property on="Intensity Chart" class="IntChart (strict)"("ZScale.MarkerVals[]"=w218) -> ()  [unwired: 2 in, 2 out]
            n135 = property on="Intensity Graph" class="IntGraph (strict)"("ZScale.MarkerVals[]"=w218) -> ()  [unwired: 2 in, 2 out]
            n136 = Bundle By Name(cluster=w217, "curr acq"=0) -> (w215:T9)
          }
          frame "reset" {
            n137 = Initialize Array(u32 0 ("element"), 0 ("dimension size")) -> (w221:u32[])
            n138 = Initialize Array(0.0 ("element"), 1024 ("dimension size"), 0 ("dimension size")) -> (w220:dbl[][])
            n139 = Bundle By Name(cluster=w222, "acq num"=w221, "signal (accum.)"=w220) -> (w219:T9)
          }
          frame "process" {
            # "transfer also trig and PD"
            n140 = Unbundle By Name(w264) -> ("acq num"=w268:u32[], "signal (accum.)"=w267:dbl[][], "curr acq"=w263:i32)
            n141 = Unbundle By Name(w228) -> ("raw data"=w281:dbl[][][], "trigger"=w280:bool[][], "raw PDs"=w244:dbl[][])
            n142 = Tick Count (ms)() -> (millisecond timer value=w274:u32)
            n143 = feedback #1() -> (w273:u32)
            n144 = feedback-in #1(w274) -> ()
            n145 = for {
              tunnel: w281 -> [w320] mode=indexing
              tunnel: w280 -> [w318] mode=indexing
              tunnel: [w319] -> w234 mode=indexing
              tunnel: [w317] -> w262 mode=indexing
              tunnel: w244 -> [w314] mode=indexing
              tunnel: [w313] -> w243 mode=indexing
              # "loop over sig. and ref."
              n146 = Equal To 0?(x="parity?") -> (x = 0?=w316:bool)
              n147 = call "check_signal_chopper_state.vi"("parity?"=w316, "PD in"=w314, "chopper"=w318, "data"=w320) -> ("PD out"=w313:dbl[], "chopper out"=w317:bool[], "data out"=w319:dbl[][])  [unwired: 5 in]
            }
            n148 = Subtract(x=w274, y=w273) -> (x-y=→"data proc. time":u32)
            n149 = Array Size(array=w268) -> (size(s)=w235:i32)
            n150 = Less Or Equal?(x="history length", y=w235) -> (x <= y?=w269:bool)
            n151 = case shown="True" w269 {
              tunnel: w268 -> [w302 w312]
              tunnel: [w302 w310] -> w265
              tunnel: w267 -> [w301 w309]
              tunnel: [w301 w308] -> w266
              tunnel: "history length" -> [_ w306]
              tunnel: w235 -> [_ w305]
              frame False {
              }
              frame True {
                n152 = Subtract(x=w306, y=w305) -> (x-y=w304:i32)
                n153 = Absolute Value(x=w304) -> (abs(x)=w303:i32)
                n154 = Delete From Array(array=w312, length=w303, index=0) -> (array with subset deleted=w310:u32[])  [unwired: 1 out]
                n155 = Delete From Array(array=w309, length=w303, index (row)=0 ("disabled index (col)")) -> (array with subset deleted=w308:dbl[][])  [unwired: 1 in, 1 out]
              }
            }
            n156 = case shown="True" "use dynamic offset?" {
              tunnel: w234 -> [_ w286]
              tunnel: [w282 w285] -> w232
              frame False {
                n157 = Build Array("baseline offset (signal)", "baseline offset (ref.)") -> (w282:dbl[])
              }
              frame True {
                n158 = for {
                  tunnel: w286 -> [w290] mode=indexing
                  tunnel: [w288] -> w285 mode=indexing
                  n159 = Index Array(array=w290, index (col)=0 ("index (row)")) -> (element=w289:dbl[])  [unwired: 1 in]
                  n160 = call-poly <vilib>:"Mean.vi"("X"=w289) -> ("mean"=w288:dbl)  [unwired: 1 out]
                }
              }
            }
            "dynamic offset" <- w232
            n161 = Index Array(array=w262) -> (element #1=w277:bool[], element #2=w276:bool[])  [unwired: 4 in]
            n162 = for {
              tunnel: w262 -> [w300] mode=indexing
              tunnel: [w296] -> w245 mode=indexing
              n163 = Decimate 1D Array(w300) -> (w299:bool[], w298:bool[])
              n164 = Equal?(x=w299, y=w298) -> (x = y?=w297:bool[])
              n165 = Or Array Elements(Boolean array=w297) -> (logical OR=w296:bool)
            }
            "skipped" <- w245
            n166 = Exclusive Or(1:w276, 2:w277) -> (0:w271:bool[])
            n167 = Index Array(array=w234) -> (element #1=w279:dbl[][], element #2=w278:dbl[][])  [unwired: 6 in]
            n168 = Or Array Elements(Boolean array=w271) -> (logical OR=→"synchronization error":bool)
            n169 = Insert Into Array(array=w262, new element=w271) -> (→"chopper out":bool[][])  [unwired: 2 in]
            n170 = Index Array(array=w232) -> (element #1=w231:dbl, element #2=w230:dbl)  [unwired: 2 in]
            n171 = Insert Into Array(array=w265, new element=w263) -> (w251:u32[])  [unwired: 1 in]
            n172 = Subtract(x=w279, y=w231) -> (x-y=w229:dbl[][])
            n173 = Subtract(x=w278, y=w230) -> (x-y=w259:dbl[][])
            n174 = call "ta_calc_diff.vi"("data in"=w229, "ref in"=w259, "Algorithm"="Algorithm", "PD values in"=w243) -> ("pumped std"=w254:dbl[], "unpumped std"=w255:dbl[], "pumped"=w239:dbl[], "unpumped"=w256:dbl[], "diff std"=w237:dbl[], "diff"=w241:dbl[], "ref std"=w250:dbl[], "ref mean"=w248:dbl[])  [unwired: 4 in]
            n175 = Select(t=w241, s="is measurement TA?", f=w239) -> (s? t:f=w240:dbl[])
            n176 = Insert Into Array(array=w266, new element=w240) -> (w252:dbl[][])  [unwired: 2 in]
            n177 = Increment(x=w263) -> (x+1=w253:i32)
            n178 = Bundle By Name(cluster=w228, "command"=data_process."plot") -> (w258:T7)
            n179 = Bundle By Name(cluster=w264, "signal std"=w237, "pumped std"=w254, "unpumped std"=w255, "pumped mean"=w239, "unpumped mean"=w256, "signal"=w241, "reference mean"=w248, "reference std"=w250, "acq num"=w251, "signal (accum.)"=w252, "curr acq"=w253) -> (w249:T9)
            n180 = case shown="False" "show reference spectrum?" {
              tunnel: w249 -> [w294 w295]
              tunnel: w239 -> [w293 _]
              tunnel: w248 -> [w292 _]
              tunnel: [w291 w295] -> w247
              frame False {
                n181 = Bundle By Name(cluster=w294, "pumped stored"=w293, "reference stored"=w292) -> (w291:T9)
              }
              frame True {
              }
            }
            n182 = Enqueue Element At Opposite End(queue=w261, element=w258, error in (no error)=w260) -> ()  [unwired: 1 in, 3 out]
          }
          frame "plot" {
            n183 = Unbundle By Name(w372) -> ("pumped mean"=w382:dbl[], "unpumped mean"=w381:dbl[], "reference mean"=w380:dbl[], "signal"=w331:dbl[], "pumped stored"=w352:dbl[], "reference stored"=w351:dbl[], "signal std"=w328:dbl[])
            n184 = Unbundle By Name(w363) -> ("wavelength"=w322:dbl[])
            n185 = Unbundle By Name(w363) -> ("wavelength"=w367:dbl[], "raw data"=w366:dbl[][][], "raw PDs"=w346:dbl[][], "trigger"=w345:bool[][])
            n186 = Add(x=w331, y=w328) -> (x+y=w332:dbl[])
            n187 = Array Size(array=w328) -> (size(s)=w327:i32)
            n188 = Subtract(x=w331, y=w328) -> (x-y=w330:dbl[])
            n189 = Bundle("wavelength"=w322, "pumped mean"=w382) -> (w385:cluster{"wavelength":dbl[], "pumped mean":dbl[]})  [unwired: 1 in]
            n190 = Bundle("wavelength"=w322, "unpumped mean"=w381) -> (w384:T14)  [unwired: 1 in]
            n191 = Bundle("wavelength"=w322, "reference mean"=w380) -> (w379:T15)  [unwired: 1 in]
            n192 = Bundle("wavelength"=w322, "signal"=w331) -> (w378:cluster{"wavelength":dbl[], "signal":dbl[]})  [unwired: 1 in]
            n193 = property on="main graph" class="XYGraph (strict)"() -> ("CrsrList"=w369:T12)  [unwired: 2 in, 2 out]
            n194 = Bundle("wavelength"=w322, "reference stored"=w351) -> (w349:T16)  [unwired: 1 in]
            n195 = Bundle("wavelength"=w322, "pumped stored"=w352) -> (w350:T17)  [unwired: 1 in]
            n196 = Initialize Array(0.0 ("element"), w327) -> (w323:dbl[])
            n197 = call "view_full_data.vi"("data"=w366, "wavelength"=w367) -> ()  [unwired: 10 in]
            n198 = call "error_anal.vi"("data"=w366, "wavelength"=w367) -> ()  [unwired: 10 in]
            n199 = for {
              tunnel: w369 -> [w419] mode=indexing
              tunnel: w367 -> [w425]
              tunnel: [w424] -> w354 mode=indexing
              tunnel: [w421] -> w355 mode=indexing
              tunnel: [w420] -> w368 mode=indexing
              n200 = Unbundle By Name(w419) -> ("Position.Y"=w424:dbl, "Position.X"=w420:dbl)
              n201 = Subtract(x=w425, y=w420) -> (x-y=w423:dbl[])
              n202 = Absolute Value(x=w423) -> (abs(x)=w422:dbl[])
              n203 = Array Max & Min(array=w422) -> (min index (indices)=w421:i32)  [unwired: 3 out]
            }
            "Cursor position (idx)" <- w355
            "Cursor position (wl)" <- w368
            n204 = Bundle("wavelength"=w322, w323) -> (w324:cluster{"wavelength":dbl[], dbl[]})  [unwired: 1 in]
            n205 = Bundle("wavelength"=w322, w332) -> (w326:cluster{"wavelength":dbl[], dbl[]})  [unwired: 1 in]
            n206 = Bundle("wavelength"=w322, w330) -> (w325:cluster{"wavelength":dbl[], dbl[]})  [unwired: 1 in]
            n207 = for {
              tunnel: [w391] -> w341 mode=indexing
              tunnel: [w396] -> w344 mode=indexing
              tunnel: i32[] [] -> [w395]
              tunnel: dbl[] [] -> [w394]
              tunnel: w346 -> [w393] mode=indexing
              tunnel: w345 -> [w392] mode=indexing
              tunnel: [w390] -> w340 mode=indexing
              tunnel: [w386] -> w333 mode=indexing
              n208 = for {
                shift-right: [w398] -> w389
                shift-left: w394 -> [w404]
                shift-right: [w403] -> w397
                shift-left: w395 -> [w402]
                tunnel: w393 -> [w400] mode=indexing
                tunnel: w392 -> [w399] mode=indexing
                i -> [w401]
                n209 = case shown="True" w399 {
                  tunnel: [w405 w412] -> w398
                  tunnel: w404 -> [w405 w411]
                  tunnel: [w406 w410] -> w403
                  tunnel: w402 -> [w406 w409]
                  tunnel: w401 -> [_ w408]
                  tunnel: w400 -> [_ w407]
                  frame False {
                  }
                  frame True {
                    n210 = Build Array (concatenate)(w409, w408) -> (w410:i32[])
                    n211 = Build Array (concatenate)(w411, w407) -> (w412:dbl[])
                  }
                }
              }
              n212 = call <vilib>:"Histogram.vi"("X"=w389) -> ("X Values"=w387:dbl[], "Histogram: h(x)"=w388:i32[])  [unwired: 7 in, 2 out]
              n213 = Bundle(w397, w389) -> (w396:cluster{i32[], dbl[]})  [unwired: 1 in]
              n214 = call <vilib>:"Std Deviation and Variance.vi"("X"=w389) -> ("mean"=w391:dbl, "standard deviation"=w390:dbl)  [unwired: 1 in, 1 out]
              n215 = Bundle("Histogram: h(x)"=w388, "X Values"=w387) -> (w386:T18)  [unwired: 1 in]
            }
            "PD" <- w344
            "PD hist" <- w333
            "PDs mean" <- w341
            "PDs std" <- w340
            n216 = Build Array(w385, w384, w379, w378, w350, w349, w324, w326, w325) -> (w357:T19)
            n217 = Unbundle By Name(w363) -> ("save flag"=w360:bool, "save type"=w362:bool[])
            n218 = local write "main graph"(w357) -> ()
            n219 = Unbundle By Name(w372) -> ("pumped std"=w377:dbl[], "unpumped std"=w376:dbl[], "reference std"=w375:dbl[], "signal"=w374:dbl[], "signal (accum.)"=w373:dbl[][])
            n220 = Index Array(array=w362, index=3) -> (element=w359:bool)
            n221 = local read "Tab Control"() -> (w383:T2)
            n222 = Or(x=w360, y=w359) -> (x .or. y?=w358:bool)
            n223 = case shown="\"y/x\"" w383 {
              tunnel: w322 -> [_ _ w436]
              tunnel: w377 -> [_ _ w435]
              tunnel: w376 -> [_ _ w434]
              tunnel: w375 -> [_ _ w433]
              tunnel: w374 -> [w426 _ _]
              tunnel: w373 -> [_ w428 _]
              frame "x/y", Default {
                n224 = Build Array(w426) -> (→"Intensity Chart":dbl[][])
              }
              frame "y/x" {
                n225 = Transpose 2D Array(2D array=w428) -> (transposed array=w431:dbl[][])
                n226 = Multiply(x=w431, y=1000.0) -> (x*y=→"Intensity Graph":dbl[][])
              }
              frame "std" {
                n227 = Bundle("wavelength"=w436, "pumped std"=w435) -> (w437:cluster{"wavelength":dbl[], "pumped std":dbl[]})  [unwired: 1 in]
                n228 = Bundle("wavelength"=w436, "unpumped std"=w434) -> (w438:T20)  [unwired: 1 in]
                n229 = Bundle("wavelength"=w436, "reference std"=w433) -> (w439:T21)  [unwired: 1 in]
                n230 = Build Array(w437, w438, w439) -> (→"std graph":T22)
              }
            }
            n231 = Array To Cluster(array=w354) -> (cluster=→"Waveform Chart":T3)
            n232 = case shown="True" w358 {
              tunnel: w365 -> [_ w416]
              tunnel: w364 -> [_ w415]
              tunnel: w363 -> [_ w414]
              frame False {
              }
              frame True {
                n233 = Bundle By Name(cluster=w414, "command"=data_process."save") -> (w418:T7)
                n234 = Enqueue Element At Opposite End(queue=w416, element=w418, error in (no error)=w415) -> ()  [unwired: 1 in, 3 out]
              }
            }
            n235 = Unbundle By Name(w372) -> ("acq num"=w371:u32[])
            n236 = First Call?() -> (First Call?: T/F=w356:bool)
            n237 = Add(x=w341, y=w340) -> (x+y=w342:dbl[])
            n238 = Subtract(x=w341, y=w340) -> (x-y=w339:dbl[])
            n239 = case shown="True" w356 {
              tunnel: w355 -> [_ _]
              frame False {
              }
              frame True {
                n240 = property on="main graph" class="XYGraph (strict)"("Cursor.Cursor X"=500.0 ("Cursor.Cursor Position:Cursor X")) -> ()  [unwired: 2 in, 2 out]
              }
            }
            n241 = Index Array(array=w339) -> (element #1=→"Tank 1 - std" →"element 3":dbl, element #2=→"Tank 2 + std":dbl)  [unwired: 2 in]
            n242 = Index Array(array=w341) -> (element #1=→"Tank 1" →"mean":dbl, element #2=→"Tank 2":dbl)  [unwired: 2 in]
            n243 = Index Array(array=w342) -> (element #1=→"Tank 1 + std" →"element 2":dbl, element #2=→"Tank 2 - std":dbl)  [unwired: 2 in]
            n244 = Index Array(array=w371) -> (element=w370:u32)  [unwired: 1 in]
            n245 = property on="Intensity Graph" class="IntGraph (strict)"("YScale.Offset"=w370) -> ()  [unwired: 2 in, 2 out]
          }
          frame "save" {
            # "this won't work atm"
            n246 = Unbundle By Name(w471) -> ("scn_step_time_dly (set) [fs]"=w441:dbl[][], "scn_step"=w463:i32, "save type"=w458:bool[], "scn_iter"=w464:i32, "wavelength"=w470:dbl[], "raw data"=w465:dbl[][][], "scn_step_time_dly (set) [fs]"=w440:dbl[][], "save path"=w460:path)  [unwired: 1 out]
            n247 = Unbundle By Name(w469) -> ("pumped mean"=w468:dbl[], "unpumped mean"=w467:dbl[], "reference mean"=w466:dbl[], "signal (accum.)"=w461:dbl[][])
            n248 = Increment(x=w463) -> (x+1=w443:i32)
            n249 = Array Size(array=w441) -> (size(s)=w447:i32[])
            n250 = Index Array(array=w441) -> (element=w450:dbl[])  [unwired: 2 in]
            n251 = Build Array("Title", "Experimenter", "Experimental parameters") -> (w451:string[])
            n252 = Index Array(array=w447) -> (element=w445:i32)  [unwired: 1 in]
            n253 = Array Size(array=w450) -> (size(s)=w462:i32)
            n254 = Index Array(array=w458, index=3) -> (element=w457:bool)
            n255 = Decrement(x=w445) -> (x-1=w446:i32)
            n256 = Equal?(x=w462, y=w443) -> (x = y?=w459:bool)
            n257 = Index Array(array=w441, index (row)=w446) -> (element=w449:dbl[])  [unwired: 1 in]
            n258 = Or(x=w459, y=w457) -> (x .or. y?=w455:bool)
            n259 = call "Remove Duplicates From 1D Array.vim"("array"=w449) -> ("array with duplicates removed"=w448:dbl[])  [unwired: 10 in]
            n260 = Array Size(array=w448) -> (size(s)=w444:i32)
            "size of dependent time scan 2" <- w444
            n261 = case shown="True" w455 {
              tunnel: w470 -> [_ w486]
              tunnel: w468 -> [_ w476]
              tunnel: w467 -> [_ _]
              tunnel: w466 -> [_ w475]
              tunnel: w465 -> [_ w477]
              tunnel: w458 -> [_ w478]
              tunnel: w464 -> [_ _]
              tunnel: w461 -> [_ w485]
              tunnel: w460 -> [_ w474]
              tunnel: w440 -> [_ w484]
              tunnel: w451 -> [_ w473]
              frame False {
              }
              frame True {
                # "crop to only the transients of current scan"
                n262 = Index Array(array=w484) -> (element=w472:dbl[])  [unwired: 2 in]
                n263 = Array Size(array=w485) -> (size(s)=w483:i32[])
                n264 = Array Size(array=w472) -> (size(s)=w480:i32)
                n265 = Index Array(array=w483) -> (element=w482:i32)  [unwired: 1 in]
                n266 = Subtract(x=w482, y=w480) -> (x-y=w481:i32)
                n267 = Array Subset(array=w485, index (row)=w481, length (row)=w480) -> (w479:dbl[][])  [unwired: 2 in]
                n268 = call "saving.vi"("file path (use dialog)"=w474, "save type"=w478, "details"=w473, "signal mean"=w476, "wavelength"=w486, "time delays"=w484, "signal (accum.)"=w479, "raw data"=w477, "reference mean"=w475) -> ()  [unwired: 7 in]
              }
            }
            n269 = Equal?(x=w444, y=w443) -> (x = y?=→"x = y?":bool)
          }
          frame "exit" {
            n270 = Release Queue(queue=w487) -> ()  [unwired: 2 in, 3 out]
          }
        }
      }
    }
    frame Enabled {
    }
  }
  n271 = while {
    shift-right: [w512] -> _
    shift-left: "_camera" -> [w513]
    tunnel: w68 -> [w492]
    tunnel: w67 -> [w511]
    shift-right: [w503] -> w128
    shift-left: "error in (no error)" -> [w505]
    shift-right: [w507] -> _
    shift-left: "stages" -> [w506]
    tunnel: w69 -> [w497]
    shift-right: [w495] -> _
    shift-left: w104 -> [w501]
    tunnel: w103 -> [w494]
    tunnel: w105 -> [w493]
    tunnel: w40 -> [_]
    tunnel: w12 -> [w491]
    tunnel: w13 -> [w490]
    stop <- w510 stop-if-true
    # "Hardware and DAQ"
    n272 = Dequeue Element(queue=w492, timeout in ms (-1)=75, error in (no error)=w511) -> (queue out=w509:refnum<queue>, element=w499:cluster{"state":T8, "value":variant}, error out=w508:errorcluster)  [unwired: 1 out]
    n273 = Unbundle(w499) -> ("state"=w498:T8, "value"=w496:variant)
    n274 = case shown="\"cam_get_bg\"" w498 {
      tunnel: w513 -> [w521 w620 w689 w721 w805 w818 w833 w865 w908 w947 w973 w1001 w1042 w1088 w1126 w1140 w1157 w1183 w1196 w1202 w1229]
      tunnel: [w520 w633 w670 w718 w803 w817 w833 w839 w912 w947 w973 w1001 w1042 w1088 w1126 w1140 w1157 w1183 w1196 w1202 w1228] -> w512
      tunnel: [_ _ _ _ _ _ _ _ _ _ _ _ _ _ _ _ _ _ _ _ w1230] -> w510
      tunnel: w509 -> [w527 w601 w695 w710 _ _ w837 _ _ _ _ w996 w1038 w1091 _ _ w1170 _ _ _ w1217]
      tunnel: w508 -> [w526 w602 w694 w711 _ _ w836 _ _ _ _ w995 w1037 w1090 _ _ w1169 _ _ _ w1216]
      tunnel: w505 -> [w529 w619 w700 w720 w800 w815 w832 w864 w913 w946 w972 w1000 w1041 w1087 w1127 w1139 w1156 w1182 w1194 w1201 w1226]
      tunnel: [w528 w631 w700 w717 w798 w814 w832 w869 w913 w946 w972 w1000 w1041 w1087 w1127 w1139 w1156 w1182 w1194 w1201 w1224] -> w504
      tunnel: [w522 w612 w699 w713 w797 w813 w831 w868 w905 w945 w959 w999 w1039 w1086 w1129 w1135 w1153 w1181 w1192 w1199 w1220] -> w507
      tunnel: w506 -> [w525 w629 w699 w716 w797 w813 w831 w868 w896 w945 w959 w999 w1039 w1086 w1129 w1135 w1153 w1181 w1192 w1199 w1223]
      tunnel: w505 -> [w524 w626 w698 w715 w796 w812 w830 w867 w902 w944 w971 w998 w1040 w1085 w1128 w1134 w1152 w1180 w1193 w1198 w1222]
      tunnel: [w523 w611 w698 w714 w796 w812 w830 w867 w904 w944 w971 w998 w1040 w1085 w1128 w1134 w1152 w1180 w1193 w1198 w1221] -> w502
      tunnel: w501 -> [w514 w627 w690 w719 w795 w811 w820 w866 w910 w943 w966 w993 w1035 w1084 w1131 w1138 w1151 w1173 w1195 w1200 w1225]
      tunnel: w497 -> [w519 w603 w691 w709 _ _ w823 _ _ _ _ w994 w1036 w1089 _ _ w1160 _ _ _ w1211]
      tunnel: w496 -> [w518 _ _ _ _ _ _ w859 w911 _ w970 _ _ _ w1125 w1136 _ w1179 _ _ _]
      tunnel: [w514 w606 w690 w704 w795 w811 w820 w866 w910 w943 w965 w991 w1034 w1092 w1130 w1137 w1150 w1173 w1195 w1200 w1207] -> w495
      tunnel: w494 -> [_ _ _ _ _ _ _ _ _ _ _ _ _ _ _ _ _ w1175 _ _ w1209]
      tunnel: w493 -> [_ _ _ _ _ _ _ _ _ _ _ _ _ _ _ _ _ w1174 _ _ w1208]
      tunnel: w491 -> [_ _ _ w702 _ _ _ _ _ _ _ _ _ _ _ _ _ _ _ _ w1205]
      tunnel: w490 -> [_ _ _ w701 _ _ _ _ _ _ _ _ _ _ _ _ _ _ _ _ _]
      frame "timeout", Default {
        w516 = TRUE ("Boolean 2")
        n275 = case shown="No Error" w529 {
          selector: w529 -> [w533 w595]
          tunnel: [w544 w595] -> w528
          tunnel: w527 -> [_ w597]
          tunnel: w526 -> [_ w596]
          tunnel: w525 -> [w541 w593]
          tunnel: w524 -> [w543 w592]
          tunnel: [w542 w592] -> w523
          tunnel: [w540 w593] -> w522
          tunnel: w521 -> [w532 w594]
          tunnel: [w545 w594] -> w520
          tunnel: w519 -> [_ w591]
          tunnel: w518 -> [_ _]
          tunnel: [FALSE TRUE ("Boolean")] -> w517
          tunnel: w516 -> [w538 w585]
          tunnel: [w537 w584] -> w515
          frame No Error {
            n276 = First Call?() -> (First Call?: T/F=w535:bool)
            n277 = case shown="False" w535 {
              tunnel: w543 -> [w552 w570]
              tunnel: [w551 w568] -> w542
              tunnel: w541 -> [w547 w565]
              tunnel: [w550 w569] -> w540
              tunnel: [w549 w567] -> w534
              tunnel: [w548 w566] -> w531
              frame False {
                n278 = Array Size(array=w547) -> (size(s)=w546:i32)
                n279 = for {
                  N: w546 -> [_]
                  shift-right: [w553] -> w551
                  shift-left: w552 -> [w556]
                  tunnel: w547 -> [w559] mode=indexing
                  tunnel: [w554] -> w550 mode=indexing
                  tunnel: [w555] -> w548 mode=indexing
                  tunnel: [w560] -> w549 mode=indexing
                  workers-P: w546 -> [_]
                  n280 = call-dynamic "check_is_moving.vi"("error in (no error)"=w556, "_stage in"=w559) -> ("error out"=w557:errorcluster, "_stage out"=w558:refnum<class "_stage.lvclass">)  [unwired: 7 in, 1 out]
                  n281 = call-dynamic "Read is moving_.vi"("error in (no error)"=w557, "_stage in"=w558) -> ("error out"=w561:errorcluster, "is moving?"=w560:bool, "_stage out"=w562:refnum<class "_stage.lvclass">)  [unwired: 7 in]
                  n282 = call-dynamic "get_curr_position.vi"("error in (no error)"=w561, "_stage in"=w562) -> ("error out"=w553:errorcluster, "readback position"=w563:dbl[], "_stage out"=w554:refnum<class "_stage.lvclass">)  [unwired: 7 in]
                  n283 = Index Array(array=w563) -> (element=w555:dbl)  [unwired: 1 in]
                }
              }
              frame True {
                # "set readback position as first stage position"
                n284 = Array Size(array=w565) -> (size(s)=w564:i32)
                n285 = for {
                  N: w564 -> [_]
                  tunnel: w565 -> [w583] mode=indexing
                  tunnel: [w574] -> w569 mode=indexing
                  tunnel: [w572] -> w567 mode=indexing
                  shift-right: [w573] -> w568
                  shift-left: w570 -> [w582]
                  tunnel: [w571] -> w566 mode=indexing
                  workers-P: w564 -> [_]
                  n286 = call-dynamic "check_is_moving.vi"("error in (no error)"=w582, "_stage in"=w583) -> ("error out"=w580:errorcluster, "Numeric"=w571:dbl, "_stage out"=w581:refnum<class "_stage.lvclass">)  [unwired: 7 in]
                  n287 = Build Array(w571) -> (w579:dbl[])
                  n288 = call-dynamic "Write pos_curr.vi"("error in (no error)"=w580, "set_pos"=w579, "_stage in"=w581) -> ("error out"=w577:errorcluster, "_stage out"=w578:refnum<class "_stage.lvclass">)  [unwired: 7 in]
                  n289 = call-dynamic "check_is_moving.vi"("error in (no error)"=w577, "_stage in"=w578) -> ("error out"=w575:errorcluster, "_stage out"=w576:refnum<class "_stage.lvclass">)  [unwired: 7 in, 1 out]
                  n290 = call-dynamic "Read is moving_.vi"("error in (no error)"=w575, "_stage in"=w576) -> ("error out"=w573:errorcluster, "is moving?"=w572:bool, "_stage out"=w574:refnum<class "_stage.lvclass">)  [unwired: 7 in]
                }
                n291 = local write "stage position(s)"(w566) -> ()
              }
            }
            "stage position(s) readback" <- w531
            n292 = Not(x=w538) -> (.not. x?=w537:bool)
            n293 = property on="trig1 level" class="Slide (strict)"() -> ("Scale.Range"=w530:T11)  [unwired: 2 in, 2 out]
            n294 = property on="Tank 1" class="Slide (strict)"("Scale.Range"=w530) -> ()  [unwired: 2 in, 2 out]
            n295 = Wait (ms)(milliseconds to wait=u32 100) -> ()  [unwired: 1 out]
            n296 = property class="_camera.lvclass"(reference=w532, error in=w533, "stage positions readback"=w531) -> (reference out=w545:refnum<class "_camera.lvclass">, error out=w544:errorcluster)
            n297 = local write "is moving?"(w534) -> ()
          }
          frame Error {
            n298 = Bundle(cluster=w591, "state"=state."stop" ("element")) -> (w589:cluster{"state":T8, "value":variant})  [unwired: 1 in]
            n299 = Enqueue Element(queue=w597, element=w589, error in (no error)=w596) -> ()  [unwired: 1 in, 3 out]
            n300 = Not(x=w585) -> (.not. x?=w584:bool)
            n301 = One Button Dialog(message="timeout caught an error", button name ("OK")="Exit and tell me what's up!") -> ()  [unwired: 1 out]
          }
        }
        "Boolean" <- w517
        n302 = local write "timed out?"(w515) -> ()
        "timed out?" <- w516
      }
      frame "hw_init" {
        n303 = flat-sequence {
          tunnel: w629 -> [w654]
          tunnel: w627 -> [w655]
          tunnel: w626 -> [w653]
          tunnel: [w651] -> w625
          tunnel: [w655] -> w624
          tunnel: [w649] -> w621
          tunnel: w620 -> [w650]
          tunnel: w619 -> [w648]
          tunnel: [w647] -> w618
          tunnel: [w652] -> w615
          tunnel: [w668] -> w623
          tunnel: [w669] -> w628
          tunnel: w625 -> [w669]
          tunnel: w624 -> [w668]
          tunnel: [w664] -> w622
          tunnel: w621 -> [w666]
          tunnel: w618 -> [w665]
          tunnel: [w663] -> w617
          tunnel: [w667] -> w616
          tunnel: w615 -> [w667]
          frame #0 {
            n304 = local read "camera config"() -> (w646:path)
            n305 = for {
              tunnel: w654 -> [w662] mode=indexing
              tunnel: [w657] -> w651 mode=indexing
              shift-right: [w656] -> w652
              shift-left: w653 -> [w661]
              i -> [w658]
              n306 = call-dynamic "set_params.vi"("_stage in"=w662, "error in (no error)"=w661) -> ("_stage out"=w660:refnum<class "_stage.lvclass">, "error out"=w659:errorcluster)  [unwired: 7 in]
              n307 = call-dynamic "Write stage num.vi"("error in (no error)"=w659, "stage num"=w658, "_stage in"=w660) -> ("error out"=w656:errorcluster, "_stage out"=w657:refnum<class "_stage.lvclass">)  [unwired: 7 in]
            }
            n308 = property class="_camera.lvclass"(reference=w650, error in=w648, "config file path"=w646) -> (reference out=w649:refnum<class "_camera.lvclass">, error out=w647:errorcluster)
          }
          frame #1 {
            n309 = call-dynamic "set_params.vi"("error in (no error)"=w665, "_camera in"=w666) -> ("error out"=w663:errorcluster, "_camera out"=w664:refnum<class "_camera.lvclass">)  [unwired: 8 in]
          }
        }
        n310 = To Variant(anything=FALSE) -> (Variant=w598:variant)
        n311 = Bundle(cluster=w603, "state"=state."cam_set_wl", "value"=w598) -> (w605:cluster{"state":T8, "value":variant})
        n312 = Enqueue Element(queue=w601, element=w605, error in (no error)=w602) -> ()  [unwired: 1 in, 3 out]
        n313 = call-dynamic "init_hw.vi"("error in (no error)"=w617, "_camera in"=w622) -> ("error out"=w632:errorcluster, "success ?"=w608:bool, "_camera out"=w634:refnum<class "_camera.lvclass">)  [unwired: 7 in]
        n314 = for {
          tunnel: w628 -> [w645] mode=indexing
          tunnel: [w644] -> w609 mode=indexing
          tunnel: [w643] -> w614 mode=indexing
          shift-right: [w642] -> w613
          shift-left: w616 -> [w641]
          n315 = call-dynamic "init_hw.vi"("error in (no error)"=w641, "_stage in"=w645) -> ("error out"=w642:errorcluster, "Boolean"=w644:bool, "_stage out"=w643:refnum<class "_stage.lvclass">)  [unwired: 7 in]
        }
        "Stage(s) initialized" <- w609
        n316 = Build Array(w608) -> (→"Camera initialised?":bool[])
        n317 = property class="_camera.lvclass"(reference=w634, error in=w632) -> (reference out=w633:refnum<class "_camera.lvclass">, error out=w631:errorcluster, "camera name and version"=→"camera name, version":string)
        n318 = Bundle By Name(cluster=w623, "command"=data_process."init") -> (w606:T7)
        n319 = for {
          tunnel: w614 -> [w640] mode=indexing
          tunnel: [w638] -> w612 mode=indexing
          shift-right: [w637] -> w611
          shift-left: w613 -> [w639]
          tunnel: [w636] -> w610 mode=indexing
          n320 = call-dynamic "Read stage name and version.vi"("error in (no error)"=w639, "_stage in"=w640) -> ("error out"=w637:errorcluster, "stage name and version"=w636:string, "_stage out"=w638:refnum<class "_stage.lvclass">)  [unwired: 7 in]
        }
        n321 = property on="stage name(s)" class="LstBox (strict)"("Item Names"=w610) -> ()  [unwired: 2 in, 2 out]
        "vi running?" <- TRUE
      }
      frame "sw_init" {
        w673 = "dataTA"
        w687 = refnum<class "_data.lvclass"> refnum  # _data.lvlibp:_data.lvclass
        w692 = bool[] [TRUE, TRUE, TRUE, FALSE]
        # "workaround for now"
        n322 = To Variant(anything=w692) -> (Variant=w693:variant)
        n323 = property on="save type" class="Arr (strict)"("Value"=w692) -> ()  [unwired: 2 in, 2 out]
        n324 = Bundle(cluster=w691, "state"=state."dat_update_save_type", "value"=w693) -> (w697:cluster{"state":T8, "value":variant})
        n325 = Enqueue Element(queue=w695, element=w697, error in (no error)=w694) -> ()  [unwired: 1 in, 3 out]
        n326 = property class="App"() -> ("App.Kind"=w685:T5)  [unwired: 2 in, 2 out]
        n327 = Equal?(x=w685, y=T5."Run Time System") -> (x = y?=w683:bool)
        n328 = Select(t="data" ("name or relative path"), s=w683, f="builds\\data" ("name or relative path")) -> (s? t:f=w680:string)
        n329 = call <vilib>:"Application Directory.vi"() -> ("Application Directory"=w686:path)
        n330 = Build Path(base path=w686, name or relative path=w680) -> (appended path=w674:path)
        n331 = Format Into String(format string="%s\\\\%s.lvlibp", w673, w673) -> (resulting string=w677:string)  [unwired: 2 in, 1 out]
        n332 = Format Into String(format string="%s.lvlibp:%s.lvclass", w673, w673) -> (resulting string=w678:string)  [unwired: 2 in, 1 out]
        n333 = Build Path(base path=w674, name or relative path=w677) -> (appended path=w679:path)
        n334 = call <vilib>:"Get Exported File Path.vi"("qualified name"=w678, "packed library path"=w679) -> ("path"=w672:path)  [unwired: 8 in, 1 out]
        n335 = call <vilib>:"Get LV Class Default Value.vi"("class path"=w672) -> ("object"=w688:refnum<class>)  [unwired: 9 in, 1 out]
        n336 = To More Specific Class(target class=w687, reference=w688) -> (specific class reference=w671:refnum<class "_data.lvclass">)  [unwired: 1 in, 1 out]
        n337 = property class="_camera.lvclass"(reference=w689, "_data.lvlibp__data.lvclass"=w671) -> (reference out=w670:refnum<class "_camera.lvclass">)  [unwired: 1 in, 1 out]
      }
      frame "cam_single_acq" {
        n338 = local read "is moving?"() -> (w712:bool[])
        n339 = Tick Count (ms)() -> (millisecond timer value=w703:u32)
        n340 = Equal To 0?(x="move stage") -> (x = 0?=w705:bool)
        n341 = Or Array Elements(Boolean array=w712) -> (logical OR=w708:bool)
        n342 = And(x=w708, y=w705) -> (x .and. y?=w707:bool)
        n343 = case shown="False" w707 {
          tunnel: w721 -> [w741 w786]
          tunnel: w720 -> [w740 w785]
          tunnel: w719 -> [w739 w781]
          tunnel: [w738 w786] -> w718
          tunnel: [w737 w785] -> w717
          tunnel: w716 -> [w729 w784]
          tunnel: w715 -> [w736 w783]
          tunnel: [w735 w783] -> w714
          tunnel: [w733 w784] -> w713
          tunnel: w711 -> [w731 w794]
          tunnel: w710 -> [w730 w793]
          tunnel: w709 -> [w732 w787]
          tunnel: [w726 w781] -> w704
          tunnel: w703 -> [w727 _]
          tunnel: w702 -> [w723 _]
          tunnel: w701 -> [w722 _]
          frame False {
            n344 = disable-structure shown="Enabled" {
              disable-tunnel: w741 -> [w764 w771]
              disable-tunnel: w740 -> [w763 w770]
              disable-tunnel: w739 -> [w762 w772]
              disable-tunnel: [w760 w771] -> w738
              disable-tunnel: [w758 w770] -> w737
              disable-tunnel: w732 -> [w755 _]
              disable-tunnel: w731 -> [w754 _]
              disable-tunnel: w730 -> [w753 _]
              disable-tunnel: [w748 w772] -> w726
              disable-tunnel: _ -> [w747 _]
              disable-tunnel: [w742 _] -> _
              disable-tunnel: w723 -> [_ w769]
              disable-tunnel: w722 -> [_ w768]
              frame Disabled {
                n345 = call-dynamic "get_single_acq.vi"("error in (no error)"=w763, "_camera in"=w764) -> ("error out"=w759:errorcluster, "trigger"=w743:dbl[][], "raw data"=w745:i32[][][], "_camera out"=w761:refnum<class "_camera.lvclass">)  [unwired: 6 in]
                n346 = property class="_camera.lvclass"(reference=w761, error in=w759) -> (reference out=w760:refnum<class "_camera.lvclass">, error out=w758:errorcluster, "wavelength"=w746:dbl[])
                n347 = Build Array("trig1 level", "trig2 level") -> (w750:dbl[])
                n348 = for {
                  tunnel: w743 -> [w767] mode=indexing
                  tunnel: [w766] -> w744 mode=indexing
                  tunnel: w750 -> [w765] mode=indexing
                  n349 = Greater?(x=w767, y=w765) -> (0:w766:bool[])
                }
                n350 = Bundle(cluster=w755, "state"=state."dat_send_to_process") -> (w757:cluster{"state":T8, "value":variant})  [unwired: 1 in]
                n351 = Enqueue Element At Opposite End(queue=w753, element=w757, error in (no error)=w754) -> ()  [unwired: 1 in, 3 out]
                n352 = Bundle By Name(cluster=w762, "command"=data_process."process", "wavelength"=w746, "raw data"=w745, "trigger"=w744, "raw PDs"=w743) -> (w748:T7)
                n353 = property class="_data.lvclass"(reference=w747, "accessors:x dimension"=w746, "accessors:raw data"=w745, "accessors:trigger"=w744, "accessors:raw PDs"=w743) -> (reference out=w742:refnum<class "_data.lvclass">)  [unwired: 1 in, 1 out]
              }
              frame Enabled {
                n354 = Wait on Occurrence(2:w768) -> ()  [unwired: 2 in, 1 out]
                n355 = flat-sequence {
                  frame #0 {
                    n356 = Random Number (0-1)() -> (number: 0 to 1=→"number (0 to 1)":dbl)
                  }
                }
                n357 = call-by-ref "Start Asynchronous Call"(reference=w769, "error in (no error)"=w770, "_camera in"=w771) -> ()  [unwired: 7 in, 6 out]
              }
            }
            n358 = Array Size(array=w729) -> (size(s)=w728:i32)
            n359 = for {
              N: w728 -> [_]
              tunnel: w729 -> [w780] mode=indexing
              tunnel: [w775] -> w734 mode=indexing
              tunnel: [w777] -> w733 mode=indexing
              shift-right: [w778] -> w735
              shift-left: w736 -> [w779]
              workers-P: w728 -> [_]
              n360 = call-dynamic "get_curr_position.vi"("error in (no error)"=w779, "_stage in"=w780) -> ("error out"=w778:errorcluster, "readback position"=w776:dbl[], "_stage out"=w777:refnum<class "_stage.lvclass">)  [unwired: 7 in]
              n361 = Index Array(array=w776) -> (element=w775:dbl)  [unwired: 1 in]
            }
            n362 = local write "stage position(s) readback"(w734) -> ()
            n363 = flat-sequence {
              tunnel: w726 -> [_]
              tunnel: [w774] -> w725
              frame #0 {
                n364 = Tick Count (ms)() -> (millisecond timer value=w774:u32)
              }
            }
            n365 = Subtract(x=w725, y=w727) -> (x-y=→"single acq. time":u32)
          }
          frame True {
            # "need to reverse order when enqueuing at opposite end !!!!!!"
            n366 = Bundle(cluster=w787, "state"=state."cam_single_acq") -> (w792:cluster{"state":T8, "value":variant})  [unwired: 1 in]
            n367 = Enqueue Element At Opposite End(queue=w793, element=w792, error in (no error)=w794) -> (queue out=w789:refnum<queue>, error out=w788:errorcluster)  [unwired: 1 in, 1 out]
            n368 = Bundle(cluster=w787, "state"=state."timeout") -> (w790:cluster{"state":T8, "value":variant})  [unwired: 1 in]
            n369 = Enqueue Element At Opposite End(queue=w789, element=w790, error in (no error)=w788) -> ()  [unwired: 1 in, 3 out]
          }
        }
      }
      frame "cam_get_bg" {
        n370 = call-dynamic "get_single_acq.vi"("error in (no error)"=w800, "_camera in"=w805) -> ("error out"=w799:errorcluster, "raw data"=w802:i32[][][], "_camera out"=w804:refnum<class "_camera.lvclass">)  [unwired: 6 in, 1 out]
        n371 = for {
          tunnel: [w808] -> w801 mode=indexing
          tunnel: w802 -> [w806] mode=indexing
          n372 = Transpose 2D Array(2D array=w806) -> (transposed array=w807:i32[][])
          n373 = for {
            tunnel: w807 -> [w810] mode=indexing
            tunnel: [w809] -> w808 mode=indexing
            n374 = call-poly <vilib>:"Mean.vi"("X"=w810) -> ("mean"=w809:dbl)  [unwired: 1 out]
          }
        }
        n375 = property class="_camera.lvclass"(reference=w804, error in=w799, "background"=w801) -> (reference out=w803:refnum<class "_camera.lvclass">, error out=w798:errorcluster)
      }
      frame "cam_rst_bg" {
        n376 = property class="_camera.lvclass"(reference=w818, error in=w815, "background"=i32[][] []) -> (reference out=w817:refnum<class "_camera.lvclass">, error out=w814:errorcluster)
      }
      frame "cam_cnt_acq" {
        # "need to make sure that safe flag is false"
        n377 = Bundle(cluster=w823, "state"=state."cam_single_acq") -> (w829:cluster{"state":T8, "value":variant})  [unwired: 1 in]
        n378 = Enqueue Element(queue=w837, element=w829, error in (no error)=w836) -> (queue out=w835:refnum<queue>, error out=w834:errorcluster)  [unwired: 1 in, 1 out]
        n379 = Bundle(cluster=w823, "state"=state."timeout" ("element")) -> (w827:cluster{"state":T8, "value":variant})  [unwired: 1 in]
        n380 = Enqueue Element(queue=w835, element=w827, error in (no error)=w834) -> (queue out=w824:refnum<queue>, error out=w825:errorcluster)  [unwired: 1 in, 1 out]
        n381 = property on="history length" class="DigNum (strict)"("Value"=30 ("history length")) -> ()  [unwired: 2 in, 2 out]
        n382 = Bundle(cluster=w823, "state"=state."cam_cnt_acq") -> (w826:cluster{"state":T8, "value":variant})  [unwired: 1 in]
        n383 = Enqueue Element(queue=w824, element=w826, error in (no error)=w825) -> ()  [unwired: 1 in, 3 out]
      }
      frame "cam_set_wl" {
        # "Hartmann dispersion formula:\nd(\\lambda) = a1 + a2 / (pix - a3)"
        n384 = Variant To Data(type=TRUE, Variant=w859) -> (data=w858:bool)  [unwired: 1 in, 1 out]
        n385 = property class="_camera.lvclass"(reference=w865, error in=w864) -> (reference out=w842:refnum<class "_camera.lvclass">, "wavelength"=w846:dbl[])  [unwired: 1 out]
        n386 = Array Size(array=w846) -> (size(s)=w845:i32)
        n387 = for {
          N: w845 -> [_]
          tunnel: [w870] -> w844 mode=indexing
          i -> [w870]
        }
        n388 = case shown="True" w858 {
          tunnel: [w874 w887] -> w853
          tunnel: [w874 w875] -> w850
          tunnel: [w874 w890] -> w838
          tunnel: [w874 w886] -> w860
          tunnel: "pixel/index" -> [_ w878]
          tunnel: "wavelength \n(calibration value)" -> [_ w877]
          tunnel: T23 {"model"="a1+a2/(x-a3)", "Parameters"=["a1", "a2", "a3"], "x"="x"} ("model description") -> [_ w876]
          tunnel: w844 -> [w874 w875]
          frame False {
          }
          frame True {
            n389 = Sort 1D Array(array=w877) -> (sorted array=w889:dbl[])
            n390 = Sort 1D Array(array=w878) -> (sorted array=w887:u16[])
            n391 = case shown="True" "mirror?" {
              tunnel: w889 -> [w891 w893]
              tunnel: [w891 w892] -> w886
              frame False {
              }
              frame True {
                n392 = Reverse 1D Array(array=w893) -> (reversed array=w892:dbl[])
              }
            }
            n393 = call-poly <vilib>:"Nonlinear Curve Fit.vi"("Y"=w886, "initial parameters"="initial parameters", "X"=w887, "model description"=w876) -> ("best fit parameters"=w884:dbl[])  [unwired: 7 in, 4 out]
            "best fit parameters" <- w884
            n394 = Index Array(array=w884) -> (element #1=w883:dbl, element #2=w882:dbl, element #3=w880:dbl)  [unwired: 3 in]
            n395 = Subtract(x=w875, y=w880) -> (x-y=w881:dbl[])
            n396 = Divide(x=w882, y=w881) -> (x/y=w879:dbl[])
            n397 = Add(x=w883, y=w879) -> (x+y=w890:dbl[])
          }
        }
        n398 = for {
          tunnel: "pixel/index" -> [w873] mode=indexing
          tunnel: w838 -> [w872]
          tunnel: [w871] -> w856 mode=indexing
          n399 = Index Array(array=w872, index=w873) -> (element=w871:dbl)
        }
        "wavelength (fitted)" <- w856
        n400 = property class="_camera.lvclass"(reference=w842, "wavelength"=w838) -> (reference out=w840:refnum<class "_camera.lvclass">, error out=w869:errorcluster)  [unwired: 1 in]
        n401 = property class="_camera.lvclass"(reference=w840) -> ("_data.lvlibp__data.lvclass"=w843:refnum<class "_data.lvclass">)  [unwired: 1 in, 2 out]
        n402 = property class="_data.lvclass"(reference=w843, "accessors:x dimension"=w838) -> (reference out=w841:refnum<class "_data.lvclass">)  [unwired: 1 in, 1 out]
        n403 = Subtract(x="wavelength \n(calibration value)", y=w856) -> (x-y=w855:dbl[])
        n404 = Subtract(x=w838, y=w838) -> (x-y=w852:dbl[])
        n405 = Bundle(w853, w860) -> (w863:cluster{i32[], dbl[]})  [unwired: 1 in]
        n406 = Bundle(w850, w838) -> (w862:cluster{i32[], dbl[]})  [unwired: 1 in]
        n407 = Bundle("pixel/index"="pixel/index", w855) -> (w854:cluster{"pixel/index":u16[], dbl[]})  [unwired: 1 in]
        n408 = Bundle(w850, w852) -> (w851:cluster{i32[], dbl[]})  [unwired: 1 in]
        n409 = property class="_camera.lvclass"(reference=w840, "_data.lvlibp__data.lvclass"=w841) -> (reference out=w839:refnum<class "_camera.lvclass">)  [unwired: 1 in, 1 out]
        n410 = Build Array(w863, w862, w854, w851) -> (→"wavelength fit":cluster{"pixel/index":i32[], dbl[]}[])
      }
      frame "stg_set_pos" {
        # "parallel execution of for loop\nto address stages more or less\nsimultaneously"
        # "parallel execution of for loop"
        # "find out which stage was moved"
        n411 = property class="_camera.lvclass"(reference=w908) -> (reference out=w907:refnum<class "_camera.lvclass">, "stage positions"=w906:dbl[])  [unwired: 1 in, 1 out]
        n412 = Array Size(array=w896) -> (size(s)=w895:i32)
        n413 = Variant To Data(type=dbl[] [], Variant=w911) -> (data=w903:dbl[])  [unwired: 1 in, 1 out]
        n414 = for {
          N: w895 -> [_]
          tunnel: w896 -> [w920] mode=indexing
          tunnel: [w916] -> w901 mode=indexing
          shift-right: [w915] -> w900
          shift-left: w902 -> [w919]
          tunnel: [w914] -> w899 mode=indexing
          workers-P: w895 -> [_]
          n415 = call-dynamic "check_is_moving.vi"("error in (no error)"=w919, "_stage in"=w920) -> ("error out"=w917:errorcluster, "_stage out"=w918:refnum<class "_stage.lvclass">)  [unwired: 7 in, 1 out]
          n416 = call-dynamic "Read is moving_.vi"("error in (no error)"=w917, "_stage in"=w918) -> ("error out"=w915:errorcluster, "is moving?"=w914:bool, "_stage out"=w916:refnum<class "_stage.lvclass">)  [unwired: 7 in]
        }
        n417 = for {
          tunnel: w903 -> [w942] mode=indexing
          tunnel: w906 -> [w940]
          tunnel: [w941] -> w898 mode=indexing
          i -> [w939]
          n418 = Index Array(array=w940, index=w939) -> (element=w938:dbl)
          n419 = Not Equal?(x=w942, y=w938) -> (x != y?=w941:bool)
        }
        n420 = Or(x=w898, y=w899) -> (x .or. y?=w897:bool[])
        "is moving?" <- w897
        n421 = property on="stage position(s)" class="Arr (strict)"("Value"=w903) -> ()  [unwired: 2 in, 2 out]
        n422 = property class="_camera.lvclass"(reference=w907, "stage positions"=w903) -> (reference out=w912:refnum<class "_camera.lvclass">)  [unwired: 1 in, 1 out]
        n423 = Array Size(array=w901) -> (size(s)=w894:i32)
        n424 = for {
          N: w894 -> [_]
          tunnel: w901 -> [w929] mode=indexing
          tunnel: w897 -> [w923]
          tunnel: [w928] -> w905 mode=indexing
          shift-right: [w927] -> w904
          shift-left: w900 -> [w926]
          tunnel: w903 -> [w925]
          workers-P: w894 -> [_]
          i -> [w922]
          n425 = Index Array(array=w925, index=w922) -> (element=w924:dbl)
          n426 = Index Array(array=w923, index=w922) -> (element=w921:bool)
          n427 = case shown="True" w921 {
            tunnel: w929 -> [w931 w937]
            tunnel: [w931 w935] -> w928
            tunnel: [w930 w933] -> w927
            tunnel: w926 -> [w930 w934]
            tunnel: w924 -> [_ w932]
            frame False {
            }
            frame True {
              n428 = Build Array(w932) -> (w936:dbl[])
              n429 = call-dynamic "set_new_position.vi"("error in (no error)"=w934, "set_pos"=w936, "_stage in"=w937) -> ("error out"=w933:errorcluster, "_stage out"=w935:refnum<class "_stage.lvclass">)  [unwired: 7 in]
            }
          }
        }
        "Stage objects" <- w905
      }
      frame "stg_home" {
      }
      frame "scn_load_step_file" {
        n430 = Variant To Data(type=path "", Variant=w970) -> (data=w968:path)  [unwired: 1 in, 1 out]
        n431 = call-poly <vilib>:"Read Delimited Spreadsheet.vi"("file path (dialog if empty)"=w968, "transpose? (F)"=TRUE) -> ("all rows"=w948:dbl[][])  [unwired: 8 in, 5 out]
        n432 = Bundle By Name(cluster=w966, "scn_step_time_dly (set) [fs]"=w948) -> (w965:T7)
        n433 = Transpose 2D Array(2D array=w948) -> (transposed array=w951:dbl[][])
        "timesteps loaded from file" <- w951
        n434 = Array Size(array=w951) -> (size(s)=w954:i32[])
        n435 = Index Array(array=w951, index (col)=0 ("index (row)")) -> (element=w950:dbl[])  [unwired: 1 in]
        n436 = Index Array(array=w954, index=1) -> (element=w953:i32)
        n437 = case shown="1" w953 {
          tunnel: w950 -> [_ w974]
          frame 0, Default {
          }
          frame 1 {
            "Waveform Graph" <- w974
          }
        }
        n438 = Array Size(array=w948) -> (size(s)=w961:i32[])
        n439 = Array Size(array=w959) -> (size(s)=w957:i32)
        n440 = Index Array(array=w961) -> (element=w958:i32)  [unwired: 1 in]
        n441 = Decrement(x=w958) -> (x-1=w960:i32)
        n442 = Greater?(x=w958, y=w957) -> (0:w956:bool)
        n443 = Index Array(array=w948, index (row)=w960) -> (element=w964:dbl[])  [unwired: 1 in]
        n444 = for {
          tunnel: w948 -> [w977] mode=indexing
          tunnel: [w975] -> w955 mode=indexing
          n445 = call "Remove Duplicates From 1D Array.vim"("array"=w977) -> ("array with duplicates removed"=w976:dbl[])  [unwired: 10 in]
          n446 = Array Size(array=w976) -> (size(s)=w975:i32)
        }
        "Array" <- w955
        n447 = call "Remove Duplicates From 1D Array.vim"("array"=w964) -> ("array with duplicates removed"=w963:dbl[])  [unwired: 10 in]
        n448 = case shown="True" w956 {
          frame False {
          }
          frame True {
            n449 = One Button Dialog(message="Be careful, timestep file dimension exceeds number of stages.", button name ("OK")="\"I like to live dangerously!\"") -> ()  [unwired: 1 out]
          }
        }
        n450 = Array Size(array=w963) -> (size(s)=→"size of dependent time scan":i32)
      }
      frame "scn_init" {
        w980 = 0 ("scn_iter")
        n451 = Unbundle By Name(w993) -> ("scn_step_time_dly (set) [fs]"=w986:dbl[][])
        n452 = property on="cont acq" class="Bool (strict)"("Value"=FALSE ("cont acq")) -> ()  [unwired: 2 in, 2 out]
        n453 = for {
          tunnel: w986 -> [w1004] mode=indexing
          tunnel: [w1002] -> w985 mode=indexing
          n454 = call "Remove Duplicates From 1D Array.vim"("array"=w1004) -> ("array with duplicates removed"=w1003:dbl[])  [unwired: 10 in]
          n455 = Array Size(array=w1003) -> (size(s)=w1002:i32)
        }
        n456 = Index Array(array=w985) -> (element=w984:i32)  [unwired: 1 in]
        n457 = Empty Array?(array=w986) -> (empty?=w997:bool)
        n458 = case shown="False" w997 {
          tunnel: w996 -> [w1010 w1019]
          tunnel: w995 -> [w1009 w1018]
          tunnel: w994 -> [w1008 w1013]
          tunnel: w984 -> [w1007 _]
          frame False {
            n459 = Add(x=w1007, y=10) -> (x+y=w1006:i32)
            n460 = property on="history length" class="DigNum (strict)"("Value"=w1006) -> ()  [unwired: 2 in, 2 out]
            n461 = Bundle(cluster=w1008, "state"=state."scn_next_step") -> (w1012:cluster{"state":T8, "value":variant})  [unwired: 1 in]
            n462 = Enqueue Element(queue=w1010, element=w1012, error in (no error)=w1009) -> ()  [unwired: 1 in, 3 out]
          }
          frame True {
            n463 = Bundle(cluster=w1013, "state"=state."scn_load_step_file") -> (w1021:cluster{"state":T8, "value":variant})  [unwired: 1 in]
            n464 = Enqueue Element(queue=w1019, element=w1021, error in (no error)=w1018) -> (queue out=w1015:refnum<queue>, error out=w1014:errorcluster)  [unwired: 1 in, 1 out]
            n465 = Bundle(cluster=w1013, "state"=state."scn_init") -> (w1017:cluster{"state":T8, "value":variant})  [unwired: 1 in]
            n466 = Enqueue Element(queue=w1015, element=w1017, error in (no error)=w1014) -> ()  [unwired: 1 in, 3 out]
          }
        }
        n467 = local read "N scans"() -> (w990:u16)
        n468 = call "create_save_dir_and_fn.vi"("scn_iter"=w980, "sample"="sample", "Experiment"="Experiment", "data folder"="data folder") -> ("Path"=w981:path)  [unwired: 7 in]
        n469 = property on="progress" class="Slide (strict)"("Scale.Maximum"=w990, "Scale.Minimum"=0.0 ("Scale.Range:Minimum")) -> ()  [unwired: 2 in, 2 out]
        n470 = Bundle By Name(cluster=w993, "scn_step"=-1, "save path"=w981, "scn_iter"=w980) -> (w991:T7)
        n471 = local write "current scan"(w980) -> ()
      }
      frame "scn_next_step" {
        n472 = Unbundle By Name(w1035) -> ("scn_step_time_dly (set) [fs]"=w1026:dbl[][], "scn_step"=w1022:i32, "scn_iter"=w1031:i32)
        n473 = Index Array(array=w1026) -> (element=w1029:dbl[])  [unwired: 2 in]
        n474 = local read "t0 position(s)"() -> (w1030:dbl[])
        n475 = Array Size(array=w1029) -> (size(s)=w1028:i32)
        n476 = Increment(x=w1022) -> (x+1=w1027:i32)
        "scan progress" <- w1027
        n477 = Add(x=w1031, y=0.5) -> (x+y=→"progress":dbl)
        n478 = Increment(x=w1031) -> (x+1=→"current scan":i32)
        n479 = Greater?(x=w1028, y=w1027) -> (0:w1033:bool)
        n480 = property on="scan progress" class="Slide (strict)"("Scale.Maximum"=w1028, "Scale.Minimum"=0.0 ("Scale.Range:Minimum")) -> ()  [unwired: 2 in, 2 out]
        n481 = case shown="False" w1033 {
          tunnel: w1038 -> [w1048 w1080]
          tunnel: w1037 -> [w1047 w1079]
          tunnel: w1036 -> [w1046 w1065]
          tunnel: w1035 -> [w1044 w1063]
          tunnel: [w1044 w1062] -> w1034
          tunnel: w1026 -> [_ w1059]
          tunnel: w1027 -> [_ w1050]
          tunnel: w1030 -> [_ w1060]
          tunnel: [w1043 w1050] -> _
          tunnel: w1022 -> [w1043 _]
          frame False {
            n482 = Bundle(cluster=w1046, "state"=state."scn_next_iter") -> (w1049:cluster{"state":T8, "value":variant})  [unwired: 1 in]
            n483 = Enqueue Element(queue=w1048, element=w1049, error in (no error)=w1047) -> ()  [unwired: 1 in, 3 out]
          }
          frame True {
            n484 = Boolean To (0,1)(Boolean="reversed?") -> (0, 1=w1056:i16[])
            n485 = Multiply(x=w1056, y=2) -> (x*y=w1054:i32[])
            n486 = Index Array(array=w1059, index (col)=w1050) -> (element=w1051:dbl[])  [unwired: 1 in]
            n487 = Subtract(x=w1054, y=1) -> (x-y=w1052:i32[])
            n488 = Multiply(x=w1052, y=w1051) -> (x*y=w1058:dbl[])
            n489 = Subtract(x=w1060, y=w1058) -> (x-y=w1061:dbl[])
            n490 = Bundle(cluster=w1065, "state"=state."stg_set_pos", "value"=w1061) -> (w1078:cluster{"state":T8, "value":variant})
            n491 = Enqueue Element(queue=w1080, element=w1078, error in (no error)=w1079) -> (queue out=w1075:refnum<queue>, error out=w1074:errorcluster)  [unwired: 1 in, 1 out]
            n492 = Bundle By Name(cluster=w1063, "scn_step"=w1050) -> (w1062:T7)
            n493 = Bundle(cluster=w1065, "state"=state."cam_single_acq") -> (w1076:cluster{"state":T8, "value":variant})  [unwired: 1 in]
            n494 = Enqueue Element(queue=w1075, element=w1076, error in (no error)=w1074) -> (queue out=w1071:refnum<queue>, error out=w1070:errorcluster)  [unwired: 1 in, 1 out]
            n495 = Bundle(cluster=w1065, "state"=state."timeout") -> (w1072:cluster{"state":T8, "value":variant})  [unwired: 1 in]
            n496 = Enqueue Element(queue=w1071, element=w1072, error in (no error)=w1070) -> (queue out=w1067:refnum<queue>, error out=w1066:errorcluster)  [unwired: 1 in, 1 out]
            n497 = Bundle(cluster=w1065, "state"=state."scn_next_step") -> (w1068:cluster{"state":T8, "value":variant})  [unwired: 1 in]
            n498 = Enqueue Element(queue=w1067, element=w1068, error in (no error)=w1066) -> ()  [unwired: 1 in, 3 out]
          }
        }
      }
      frame "scn_next_iter" {
        n499 = Unbundle By Name(w1084) -> ("save path"=w1083:path, "scn_iter"=w1082:i32)
        n500 = Unbundle By Name(w1084) -> ("scn_iter"=w1093:i32)
        n501 = Decrement(x="N scans") -> (x-1=w1081:u16)
        n502 = Less?(x=w1093, y=w1081) -> (x < y?=w1094:bool)
        n503 = case shown="False" w1094 {
          tunnel: w1084 -> [w1099 w1122]
          tunnel: [w1099 w1120] -> w1092
          tunnel: w1091 -> [w1101 w1117]
          tunnel: w1090 -> [w1100 w1116]
          tunnel: w1089 -> [_ w1115]
          tunnel: w1083 -> [_ w1114]
          tunnel: w1082 -> [w1097 w1104]
          frame False {
            n504 = Increment(x=w1097) -> (x+1=w1096:i32)
            n505 = Flush Queue(queue=w1101, error in (no error)=w1100) -> ()  [unwired: 3 out]
            n506 = local write "progress"(w1096) -> ()
            n507 = property on="scan" class="Bool (strict)"("Value"=FALSE ("scan")) -> ()  [unwired: 2 in, 2 out]
          }
          frame True {
            n508 = Strip Path(path=w1114) -> (stripped path=w1105:path, name=w1109:string)
            n509 = Increment(x=w1104) -> (x+1=w1103:i32)
            n510 = String Length(string=w1109) -> (length=w1113:i32)
            n511 = Bundle(cluster=w1115, "state"=state."scn_next_step") -> (w1119:cluster{"state":T8, "value":variant})  [unwired: 1 in]
            n512 = Subtract(x=w1113, y=3) -> (x-y=w1111:i32)
            n513 = String Subset(string=w1109, length (rest)=w1111) -> (substring=w1110:string)  [unwired: 1 in]
            n514 = Enqueue Element(queue=w1117, element=w1119, error in (no error)=w1116) -> ()  [unwired: 1 in, 3 out]
            n515 = Format Into String(format string="%03d", w1103) -> (resulting string=w1107:string)  [unwired: 2 in, 1 out]
            n516 = Concatenate Strings(w1110, w1107) -> (w1106:string)
            n517 = Build Path(base path=w1105, name or relative path=w1106) -> (appended path=w1102:path)
            n518 = Bundle By Name(cluster=w1122, "scn_step"=-1, "save path"=w1102, "scn_iter"=w1103) -> (w1120:T7)
          }
        }
      }
      frame "dat_update_save_flag" {
        n519 = Variant To Data(type=FALSE, Variant=w1125) -> (data=w1123:bool)  [unwired: 1 in, 1 out]
        n520 = Bundle By Name(cluster=w1131, "save flag"=w1123) -> (w1130:T7)
      }
      frame "dat_update_save_type" {
        n521 = Variant To Data(type=bool[] [], Variant=w1136) -> (data=w1132:bool[])  [unwired: 1 in, 1 out]
        n522 = Bundle By Name(cluster=w1138, "save type"=w1132) -> (w1137:T7)
      }
      frame "dat_save_raw" {
        n523 = To Variant(anything=bool[] [FALSE, FALSE, FALSE, TRUE]) -> (Variant=w1168:variant)
        n524 = Bundle(cluster=w1160, "state"=state."dat_update_save_type", "value"=w1168) -> (w1171:cluster{"state":T8, "value":variant})
        n525 = local read "data folder"() -> (w1144:path)
        n526 = Enqueue Element(queue=w1170, element=w1171, error in (no error)=w1169) -> (queue out=w1164:refnum<queue>, error out=w1163:errorcluster)  [unwired: 1 in, 1 out]
        n527 = Get Date/Time In Seconds() -> (seconds since 1Jan1904=w1147:timestamp)
        n528 = Format Date/Time String(time format string (%c)="%Y%m%d", seconds (now)=w1147) -> (date/time string=w1149:string)  [unwired: 1 in]
        n529 = Build Path(base path=w1144, name or relative path=w1149) -> (appended path=w1146:path)
        n530 = Bundle(cluster=w1160, "state"=state."cam_single_acq") -> (w1165:cluster{"state":T8, "value":variant})  [unwired: 1 in]
        n531 = Enqueue Element(queue=w1164, element=w1165, error in (no error)=w1163) -> (queue out=w1159:refnum<queue>, error out=w1158:errorcluster)  [unwired: 1 in, 1 out]
        n532 = Build Path(base path=w1146, name or relative path="raw_acquisition") -> (appended path=w1143:path)
        n533 = Build Path(base path=w1143, name or relative path="raw") -> (appended path=w1141:path)
        n534 = Unbundle By Name(w1151) -> ("save type"=w1155:bool[])
        n535 = Bundle By Name(cluster=w1151, "save path"=w1141) -> (w1150:T7)
        n536 = To Variant(anything=w1155) -> (Variant=w1154:variant)
        n537 = Bundle(cluster=w1160, "state"=state."dat_update_save_type", "value"=w1154) -> (w1161:cluster{"state":T8, "value":variant})
        n538 = Enqueue Element(queue=w1159, element=w1161, error in (no error)=w1158) -> ()  [unwired: 1 in, 3 out]
      }
      frame "dat_send_to_process" {
        n539 = Variant To Data(type=TRUE, Variant=w1179) -> (data=w1177:bool, error out=w1176:errorcluster)  [unwired: 1 in]
        n540 = case shown="No Error" w1176 {
          tunnel: w1177 -> [w1184 _]
          frame No Error {
            n541 = case shown="False" w1184 {
              frame False {
              }
              frame True {
              }
            }
          }
          frame Error {
          }
        }
        n542 = Enqueue Element(queue=w1175, element=w1173, error in (no error)=w1174) -> ()  [unwired: 1 in, 3 out]
      }
      frame "aux_save_wl_to_ini" {
        n543 = call <vilib>:"Application Directory.vi"() -> ("Application Directory"=w1191:path)
        n544 = local read "wavelength \n(calibration value)"() -> (w1188:dbl[])
        n545 = Build Path(base path=w1191, name or relative path="cameras\\spectral_calibration.ini") -> (appended path=w1186:path)
        n546 = local read "best fit parameters"() -> (w1189:dbl[])
        n547 = local read "pixel/index"() -> (w1185:u16[])
        n548 = call "save_wl_to_config.vi"("wavelength \n(calibration value)"=w1188, "best fit parameters"=w1189, "appended path"=w1186, "pix"=w1185) -> ("error out"=w1187:errorcluster)  [unwired: 7 in]
        n549 = call <vilib>:"Simple Error Handler.vi"("error in (no error)"=w1187) -> ()  [unwired: 4 in, 5 out]
      }
      frame "aux_center_cursor" {
        n550 = property on="main graph" class="XYGraph (strict)"() -> ("CrsrList"=w1197:T12)  [unwired: 2 in, 2 out]
        n551 = for {
          tunnel: w1197 -> [_] mode=indexing
          i -> [w1203]
          n552 = property on="main graph" class="XYGraph (strict)"("Active Cursor"=w1203, "Cursor.Cursor X"=500.0 ("Cursor.Cursor Position:Cursor X")) -> ()  [unwired: 2 in, 2 out]
        }
      }
      frame "stop" {
        w1230 = TRUE
        n553 = for {
          tunnel: w1223 -> [w1235] mode=indexing
          tunnel: [w1232] -> w1220 mode=indexing
          shift-right: [w1233] -> w1221
          shift-left: w1222 -> [w1234]
          n554 = call-dynamic "close_hw.vi"("error in (no error)"=w1234, "_stage in"=w1235) -> ("error out"=w1233:errorcluster, "_stage out"=w1232:refnum<class "_stage.lvclass">)  [unwired: 8 in]
        }
        n555 = Bundle(cluster=w1211, "state"=state."dat_send_to_process", "value"=TRUE) -> (w1213:cluster{"state":T8, "value":variant})
        n556 = Enqueue Element(queue=w1217, element=w1213, error in (no error)=w1216) -> (queue out=w1214:refnum<queue>, error out=w1215:errorcluster)  [unwired: 1 in, 1 out]
        n557 = call-dynamic "release_hw.vi"("error in (no error)"=w1226, "_camera in"=w1229) -> ("error out"=w1224:errorcluster, "_camera out"=w1228:refnum<class "_camera.lvclass">)  [unwired: 8 in]
        n558 = Release Queue(queue=w1214, error in (no error)=w1215) -> ()  [unwired: 1 in, 3 out]
        n559 = Close Reference(reference=w1205) -> ()  [unwired: 1 in, 1 out]
        n560 = Bundle By Name(cluster=w1225, "command"=data_process."exit") -> (w1207:T7)
        n561 = Build Array(FALSE ("camera initialized?")) -> (w1218:bool[])
        n562 = Enqueue Element(queue=w1209, element=w1207, error in (no error)=w1208) -> ()  [unwired: 1 in, 3 out]
        n563 = local write "Stage(s) initialized"(bool[] [FALSE] ("Stage(s) initialized")) -> ()
        n564 = local write "Camera initialised?"(w1218) -> ()
        n565 = Not(x=w1230) -> (.not. x?=w1231:bool)
        n566 = local write "vi running?"(w1231) -> ()
      }
    }
    n567 = Merge Errors(w504, w502) -> (w503:errorcluster)
  }
  n568 = while {
    shift-right: [w1248] -> _
    shift-left: w34 -> [w1247]
    tunnel: w13 -> [w1245]
    tunnel: w12 -> [w1244]
    shift-right: [w1242] -> _
    shift-left: w11 -> [w1241]
    stop <- w1237 stop-if-true
    n569 = call-by-ref "Wait On Asynchronous Call"(reference=w1244) -> (error out=w1240:errorcluster, "_camera out"=w1243:refnum<class "_camera.lvclass">)  [unwired: 9 in, 4 out]
    n570 = Unbundle By Name(w1240) -> ("code"=w1239:i32)
    n571 = Equal?(x=w1239, y=123) -> (x = y?=w1236:bool)
    "t/out" <- w1236
    n572 = case shown="False" w1236 {
      tunnel: [w1258 w1294] -> w1248
      tunnel: w1247 -> [w1257 w1299]
      tunnel: [w1256 TRUE] -> w1246
      tunnel: w1245 -> [w1255 _]
      tunnel: w1240 -> [w1254 _]
      tunnel: w1243 -> [w1253 _]
      tunnel: [w1252 w1295] -> w1242
      tunnel: w1241 -> [w1251 w1298]
      tunnel: [w1250 _] -> w1237
      tunnel: w1236 -> [w1249 _]
      frame False {
        n573 = case shown="No Error" w1254 {
          tunnel: [w1263 refnum<class "_data.lvclass"> refnum ("_data out")] -> w1258
          tunnel: w1257 -> [w1260 _]
          tunnel: [TRUE FALSE] -> w1256
          tunnel: w1255 -> [w1266 _]
          tunnel: w1253 -> [w1265 _]
          tunnel: w1251 -> [w1264 _]
          tunnel: [w1262 errorcluster {"status"=FALSE, "code"=0, "source"=""} ("error out")] -> w1252
          tunnel: [_ TRUE] -> w1250
          tunnel: w1249 -> [w1261 _]
          frame No Error {
            n574 = Set Occurrence(w1266) -> ()
            n575 = property class="_camera.lvclass"(reference=w1265) -> ("_data.lvlibp__data.lvclass"=w1259:refnum<class "_data.lvclass">)  [unwired: 1 in, 2 out]
            n576 = Random Number (0-1)() -> (number: 0 to 1=→"number (0 to 1) 2":dbl)
            n577 = disable-structure shown="Enabled" {
              disable-tunnel: w1259 -> [w1279 w1286]
              disable-tunnel: w1260 -> [w1278 w1287]
              disable-tunnel: w1264 -> [w1277 w1284]
              disable-tunnel: [w1274 w1283] -> w1263
              disable-tunnel: [w1273 w1282] -> w1262
              disable-tunnel: w1261 -> [_ w1285]
              frame Enabled {
                n578 = call-dynamic "process.vi"("error in (no error)"=w1277, "_data.lvlib:_data.lvclass"=w1279, "_data in"=w1278) -> ("error out"=w1280:errorcluster, "_data out"=w1281:refnum<class "_data.lvclass">)  [unwired: 7 in]
                n579 = call-dynamic "params.vi"("error in (no error)"=w1280, "_data in"=w1281) -> ("error out"=w1271:errorcluster, "_data out"=w1272:refnum<class "_data.lvclass">)  [unwired: 8 in]
                n580 = call-dynamic "accumulate.vi"("error in (no error)"=w1271, "_data in"=w1272) -> ("error out"=w1269:errorcluster, "_data out"=w1270:refnum<class "_data.lvclass">)  [unwired: 8 in]
                n581 = call-dynamic "visualise.vi"("error in (no error)"=w1269, "_data in"=w1270) -> ("error out"=w1275:errorcluster, "_data out"=w1276:refnum<class "_data.lvclass">)  [unwired: 8 in]
                n582 = call-dynamic "visualise_aux.vi"("error in (no error)"=w1275, "_data in"=w1276) -> ("error out"=w1273:errorcluster, "_data out"=w1274:refnum<class "_data.lvclass">)  [unwired: 8 in]
              }
              frame Disabled {
                n583 = call-dynamic "UI.vi"("error in (no error)"=w1284, "timeout?"=w1285, "_data.lvlib:_data.lvclass"=w1286, "_data in"=w1287) -> ("error out"=w1282:errorcluster, "_data out"=w1283:refnum<class "_data.lvclass">)  [unwired: 6 in]
              }
            }
          }
          frame Error {
          }
        }
      }
      frame True {
        n584 = call-dynamic "params.vi"("error in (no error)"=w1298, "_data in"=w1299) -> ("error out"=w1296:errorcluster, "_data out"=w1297:refnum<class "_data.lvclass">)  [unwired: 8 in]
        n585 = Random Number (0-1)() -> (number: 0 to 1=→"number (0 to 1) 3":dbl)
        n586 = call-dynamic "visualise.vi"("error in (no error)"=w1296, "_data in"=w1297) -> ("error out"=w1295:errorcluster, "_data out"=w1294:refnum<class "_data.lvclass">)  [unwired: 8 in]
      }
    }
    "Boolean 3" <- w1246
  }
  n587 = while {
    tunnel: w68 -> [w1304]
    tunnel: w67 -> [w1303]
    tunnel: w69 -> [w1300]
    stop <- w1302 stop-if-true
    # "Control"
    n588 = event shown="[1] \"calibrate wavelength\": Value Change" {
      selector: _ -> [_ _ _ _ _ _ _ _ _ _ _ _ _ _ _ _ _ _ _ _ _ _ _ _ _ _ _]
      dyn-events: _ -> [_ _ _ _ _ _ _ _ _ _ _ _ _ _ _ _ _ _ _ _ _ _ _ _ _ _ _]
      timeout: 10 -> [_ _ _ _ _ _ _ _ _ _ _ _ _ _ _ _ _ _ _ _ _ _ _ _ _ _ _]
      tunnel: w1304 -> [_ w1323 w1344 w1348 w1362 w1372 _ _ _ _ _ w1409 w1420 _ _ w1439 w1454 w1460 w1475 _ w1484 w1489 _ _ _ _ w1528]
      tunnel: w1303 -> [_ w1322 w1343 w1347 w1361 w1371 _ _ _ _ _ w1410 w1419 _ _ w1438 w1453 w1459 w1474 _ w1483 w1488 _ _ _ _ w1527]
      tunnel: [_ _ _ _ _ _ _ _ _ _ _ _ _ _ _ _ _ _ _ _ _ _ _ _ _ _ w1529] -> w1302
      tunnel: w1300 -> [_ w1324 w1342 w1345 w1359 w1370 _ _ _ _ _ w1408 w1418 _ _ w1440 w1452 w1462 w1476 _ w1481 w1490 _ _ _ _ w1526]
      event Timeout {
        n589 = event-data() -> ()  [unwired: 1 in, 3 out]
        n590 = local read "is measurement TA?"() -> (w1305:bool)
        n591 = case shown="False" w1305 {
          tunnel: [w1310 w1318] -> w1307
          tunnel: [w1309 w1317] -> w1306
          frame False {
            w1311 = 1000.0 ("y")
            n592 = local read "ampl"() -> (w1316:cluster{dbl, dbl})
            n593 = Unbundle(w1316) -> (w1313:dbl, w1315:dbl)
            n594 = Multiply(x=w1313, y=w1311) -> (x*y=w1312:dbl)
            n595 = Multiply(x=w1315, y=w1311) -> (x*y=w1314:dbl)
            n596 = Max & Min(x=w1312, y=w1314) -> (max(x,y)=w1310:dbl, min(x,y)=w1309:dbl)
          }
          frame True {
            n597 = Divide(x="diff", y=1.0) -> (x/y=w1318:dbl)
            n598 = Negate(x=w1318) -> (-x=w1317:dbl)
          }
        }
        n599 = property on="main graph" class="XYGraph (strict)"("ActYScl"=1 ("Active Y Scale"), "YScale.Maximum"=w1307, "YScale.Minimum"=w1306) -> ()  [unwired: 2 in, 2 out]
        n600 = property on="Intensity Chart" class="IntChart (strict)"("ZScale.Maximum"=w1307, "ZScale.Minimum"=w1306) -> ()  [unwired: 2 in, 2 out]
        n601 = property on="Intensity Graph" class="IntGraph (strict)"("ZScale.Maximum"=w1307, "ZScale.Minimum"=w1306) -> ()  [unwired: 2 in, 2 out]
      }
      event "calibrate wavelength": Value Change {
        n602 = event-data() -> ("NewVal"=w1321:bool)  [unwired: 1 in]
        n603 = case shown="False" w1321 {
          tunnel: w1324 -> [w1327 w1336]
          tunnel: w1323 -> [w1326 w1335]
          tunnel: w1322 -> [w1325 w1334]
          frame False {
            n604 = To Variant(anything=FALSE) -> (Variant=w1328:variant)
            n605 = Bundle(cluster=w1327, "state"=state."cam_set_wl" ("element"), "value"=w1328) -> (w1330:cluster{"state":T8, "value":variant})
            n606 = Enqueue Element(queue=w1326, element=w1330, error in (no error)=w1325) -> ()  [unwired: 1 in, 3 out]
          }
          frame True {
            n607 = To Variant(anything=TRUE) -> (Variant=w1332:variant)
            n608 = Bundle(cluster=w1336, "state"=state."cam_set_wl" ("element"), "value"=w1332) -> (w1337:cluster{"state":T8, "value":variant})
            n609 = Enqueue Element(queue=w1335, element=w1337, error in (no error)=w1334) -> ()  [unwired: 1 in, 3 out]
          }
        }
      }
      event "get_single_acq": Value Change {
        n610 = event-data() -> ("OldVal"=w1340:bool)  [unwired: 1 in]
        n611 = Bundle(cluster=w1342, "state"=state."cam_single_acq") -> (w1341:cluster{"state":T8, "value":variant})  [unwired: 1 in]
        n612 = Enqueue Element(queue=w1344, element=w1341, error in (no error)=w1343) -> ()  [unwired: 1 in, 3 out]
        n613 = property on="get_single_acq" class="Bool (strict)"("Value"=w1340) -> ()  [unwired: 2 in, 2 out]
      }
      event "get bg": Value Change {
        n614 = event-data() -> ("NewVal"=w1346:bool)  [unwired: 1 in]
        n615 = case shown="True" w1346 {
          tunnel: w1348 -> [w1353 w1358]
          tunnel: w1347 -> [w1352 w1357]
          tunnel: w1345 -> [w1351 w1356]
          frame False {
            n616 = Bundle(cluster=w1351, "state"=state."cam_rst_bg") -> (w1350:cluster{"state":T8, "value":variant})  [unwired: 1 in]
            n617 = Enqueue Element(queue=w1353, element=w1350, error in (no error)=w1352) -> ()  [unwired: 1 in, 3 out]
          }
          frame True {
            n618 = Bundle(cluster=w1356, "state"=state."cam_get_bg" ("element")) -> (w1354:cluster{"state":T8, "value":variant})  [unwired: 1 in]
            n619 = Enqueue Element(queue=w1358, element=w1354, error in (no error)=w1357) -> ()  [unwired: 1 in, 3 out]
          }
        }
      }
      event "cont acq": Value Change {
        n620 = event-data() -> ("NewVal"=w1360:bool)  [unwired: 1 in]
        n621 = case shown="False" w1360 {
          tunnel: w1362 -> [w1364 w1369]
          tunnel: w1361 -> [w1363 w1368]
          tunnel: w1359 -> [_ w1367]
          frame False {
            n622 = Flush Queue(queue=w1364, error in (no error)=w1363) -> ()  [unwired: 3 out]
          }
          frame True {
            n623 = Bundle(cluster=w1367, "state"=state."cam_cnt_acq") -> (w1366:cluster{"state":T8, "value":variant})  [unwired: 1 in]
            n624 = Enqueue Element(queue=w1369, element=w1366, error in (no error)=w1368) -> ()  [unwired: 1 in, 3 out]
          }
        }
      }
      event "center cursor": Value Change {
        n625 = event-data() -> ()  [unwired: 1 in, 2 out]
        n626 = Bundle(cluster=w1370, "state"=state."aux_center_cursor") -> (w1374:cluster{"state":T8, "value":variant})  [unwired: 1 in]
        n627 = Enqueue Element(queue=w1372, element=w1374, error in (no error)=w1371) -> ()  [unwired: 1 in, 3 out]
      }
      event "add cursor": Value Change {
        n628 = event-data() -> ()  [unwired: 1 in, 1 out]
        n629 = property on="main graph" class="XYGraph (strict)"() -> ("CrsrList"=w1382:T12)  [unwired: 2 in, 2 out]
        n630 = Array Size(array=w1382) -> (size(s)=w1376:i32)
        n631 = Index Array(array=w1382) -> (element=w1381:T13)  [unwired: 1 in]
        n632 = Index Array(array=u32[] [16776722, 16711680, 6618880, 16860, 12124158], index=w1376) -> (element=w1378:u32)
        n633 = Bundle By Name(cluster=w1381, "Color"=w1378) -> (w1380:T13)
        n634 = Insert Into Array(array=w1382, index=w1376, new element=w1380) -> (w1383:T12)
        n635 = property on="Waveform Chart" class="WFChart (strict)"("Active Plot"=w1376, "Plot.Visible?"=TRUE ("Plot.Visible")) -> ()  [unwired: 2 in, 2 out]
        n636 = property on="main graph" class="XYGraph (strict)"("CrsrList"=w1383, "Active Cursor"=w1376, "Cursor.LineWidth"=u8 2 ("Cursor.Line Width")) -> ()  [unwired: 2 in, 2 out]
      }
      event "remove cursor": Value Change {
        n637 = event-data() -> ()  [unwired: 1 in, 6 out]
        n638 = property on="main graph" class="XYGraph (strict)"() -> ("CrsrList"=w1387:T12)  [unwired: 2 in, 2 out]
        n639 = Array Size(array=w1387) -> (size(s)=w1386:i32)
        n640 = Greater?(x=w1386, y=1) -> (0:w1384:bool)
        n641 = case shown="True" w1384 {
          tunnel: w1387 -> [_ w1392]
          tunnel: w1386 -> [_ w1390]
          frame False {
          }
          frame True {
            n642 = Decrement(x=w1390) -> (x-1=w1388:i32)
            n643 = Delete From Array(array=w1392, index=w1388) -> (array with subset deleted=w1391:T12)  [unwired: 1 in, 1 out]
            n644 = property on="Waveform Chart" class="WFChart (strict)"("Active Plot"=w1388, "Plot.Visible?"=FALSE ("Plot.Visible")) -> ()  [unwired: 2 in, 2 out]
            n645 = property on="main graph" class="XYGraph (strict)"("CrsrList"=w1391) -> ()  [unwired: 2 in, 2 out]
          }
        }
      }
      event "camera max scale": Value Change {
        n646 = event-data() -> ("NewVal"=w1393:u16)  [unwired: 1 in]
        n647 = case shown="2" w1393 {
          tunnel: [65.535 16.384 4.096] -> w1394
          frame 0, Default {
          }
          frame 1 {
          }
          frame 2 {
          }
        }
        n648 = property on="ampl" class="Slide (strict)"("Scale.Maximum"=w1394) -> ()  [unwired: 2 in, 2 out]
      }
      event "ampl": Value Change {
        w1399 = 1000.0 ("y")
        n649 = event-data() -> ()  [unwired: 1 in, 6 out]
        n650 = Unbundle("ampl") -> (w1401:dbl, w1403:dbl)
        n651 = Multiply(x=w1401, y=w1399) -> (x*y=w1400:dbl)
        n652 = Multiply(x=w1403, y=w1399) -> (x*y=w1402:dbl)
        n653 = Max & Min(x=w1400, y=w1402) -> (max(x,y)=w1405:dbl, min(x,y)=w1404:dbl)
        n654 = property on="main graph" class="XYGraph (strict)"("ActYScl"=0 ("Active Y Scale"), "YScale.Maximum"=w1405, "YScale.Minimum"=w1404) -> ()  [unwired: 2 in, 2 out]
      }
      event "Scale.Range:Maximum": Value Change {
        n655 = event-data() -> ("NewVal"=w1407:dbl)  [unwired: 1 in, 5 out]
        n656 = property on="diff" class="Slide (strict)"("Scale.Maximum"=w1407) -> ()  [unwired: 2 in, 2 out]
      }
      event "save wl calibration to .ini": Value Change {
        n657 = event-data() -> ("OldVal"=w1413:bool)  [unwired: 1 in]
        n658 = Bundle(cluster=w1408, "state"=state."aux_save_wl_to_ini") -> (w1412:cluster{"state":T8, "value":variant})  [unwired: 1 in]
        n659 = Enqueue Element(queue=w1409, element=w1412, error in (no error)=w1410) -> ()  [unwired: 1 in, 3 out]
        n660 = property on="save wl calibration to .ini" class="Bool (strict)"("Value"=w1413) -> ()  [unwired: 2 in, 2 out]
      }
      event "stage position(s)": Value Change {
        n661 = event-data() -> ("NewVal"=w1414:dbl[])  [unwired: 1 in]
        n662 = To Variant(anything=w1414) -> (Variant=w1415:variant)
        n663 = Bundle(cluster=w1418, "state"=state."stg_set_pos", "value"=w1415) -> (w1417:cluster{"state":T8, "value":variant})
        n664 = Enqueue Element(queue=w1420, element=w1417, error in (no error)=w1419) -> ()  [unwired: 1 in, 3 out]
      }
      event "set as t0": Value Change {
        n665 = event-data() -> ("NewVal"=w1429:bool[], "OldVal"=w1421:bool[])  [unwired: 1 in]
        n666 = for {
          tunnel: w1429 -> [w1434] mode=indexing
          tunnel: w1421 -> [w1432]
          tunnel: [w1433] -> w1428 mode=indexing
          i -> [w1431]
          n667 = Index Array(array=w1432, index=w1431) -> (element=w1430:bool)
          n668 = Not Equal?(x=w1434, y=w1430) -> (x != y?=w1433:bool)
        }
        n669 = property on="stage position(s)" class="Arr (strict)"() -> ("Value"=w1424:dbl[])  [unwired: 2 in, 2 out]
        n670 = local write "set as t0"(w1421) -> ()
        n671 = Search 1D Array(1D array=w1428, element=TRUE) -> (index of element=w1423:i32)  [unwired: 1 in]
        n672 = Index Array(array=w1424, index=w1423) -> (element=w1422:dbl)
        n673 = Replace Array Subset(array="t0 position(s)", new element=w1422, index=w1423) -> (w1426:dbl[])
        n674 = property on="t0 position(s)" class="Arr (strict)"("Value"=w1426) -> ()  [unwired: 2 in, 2 out]
      }
      event "t0 position(s)": Value Change {
        n675 = event-data() -> ()  [unwired: 1 in, 6 out]
      }
      event "home stages": Value Change {
        # "find out which stage to home"
        n676 = event-data() -> ("NewVal"=w1437:bool[], "OldVal"=w1436:bool[])  [unwired: 1 in]
        n677 = for {
          tunnel: w1437 -> [w1449] mode=indexing
          tunnel: w1436 -> [w1447]
          tunnel: [w1448] -> w1444 mode=indexing
          i -> [w1446]
          n678 = Index Array(array=w1447, index=w1446) -> (element=w1445:bool)
          n679 = Not Equal?(x=w1449, y=w1445) -> (x != y?=w1448:bool)
        }
        n680 = Search 1D Array(1D array=w1444, element=TRUE) -> (index of element=w1441:i32)  [unwired: 1 in]
        n681 = Bundle(cluster=w1440, "state"=state."stg_home", "value"=w1441) -> (w1442:cluster{"state":T8, "value":variant})
        n682 = Enqueue Element(queue=w1439, element=w1442, error in (no error)=w1438) -> ()  [unwired: 1 in, 3 out]
      }
      event "time delay file": Value Change {
        n683 = event-data() -> ("NewVal"=w1451:path)  [unwired: 1 in]
        n684 = To Variant(anything=w1451) -> (Variant=w1450:variant)
        n685 = Bundle(cluster=w1452, "state"=state."scn_load_step_file", "value"=w1450) -> (w1456:cluster{"state":T8, "value":variant})
        n686 = Enqueue Element(queue=w1454, element=w1456, error in (no error)=w1453) -> ()  [unwired: 1 in, 3 out]
      }
      event "scan": Value Change {
        n687 = event-data() -> ("NewVal"=w1461:bool)  [unwired: 1 in]
        n688 = Flush Queue(queue=w1460, error in (no error)=w1459) -> (queue out=w1457:refnum<queue>, error out=w1458:errorcluster)  [unwired: 1 out]
        n689 = case shown="False" w1461 {
          tunnel: w1457 -> [_ w1464]
          tunnel: w1458 -> [_ w1463]
          tunnel: w1462 -> [_ w1469]
          frame False {
          }
          frame True {
            w1467 = 0
            n690 = Build Array(w1467, w1467) -> (w1466:i32[])
            n691 = To Variant(anything=w1466) -> (Variant=w1465:variant)
            n692 = Bundle(cluster=w1469, "state"=state."scn_init", "value"=w1465) -> (w1470:cluster{"state":T8, "value":variant})
            n693 = Enqueue Element(queue=w1464, element=w1470, error in (no error)=w1463) -> ()  [unwired: 1 in, 3 out]
          }
        }
      }
      event "save type": Value Change {
        n694 = event-data() -> ("NewVal"=w1471:bool[])  [unwired: 1 in]
        n695 = To Variant(anything=w1471) -> (Variant=w1473:variant)
        n696 = Bundle(cluster=w1476, "state"=state."dat_update_save_type", "value"=w1473) -> (w1477:cluster{"state":T8, "value":variant})
        n697 = Enqueue Element(queue=w1475, element=w1477, error in (no error)=w1474) -> ()  [unwired: 1 in, 3 out]
      }
      event "index": Value Change {
        n698 = event-data() -> ()  [unwired: 1 in, 2 out]
        n699 = Build Array("index") -> (w1478:u16[])
        n700 = property on="pixel/index" class="Arr (strict)"("Index Values"=w1478) -> ()  [unwired: 2 in, 2 out]
        n701 = property on="wavelength \n(calibration value)" class="Arr (strict)"("Index Values"=w1478) -> ()  [unwired: 2 in, 2 out]
        n702 = property on="wavelength (fitted)" class="Arr (strict)"("Index Values"=w1478) -> ()  [unwired: 2 in, 2 out]
      }
      event "save raw data": Value Change {
        n703 = event-data() -> ("OldVal"=w1485:bool)  [unwired: 1 in]
        n704 = Bundle(cluster=w1481, "state"=state."dat_save_raw") -> (w1480:cluster{"state":T8, "value":variant})  [unwired: 1 in]
        n705 = property on="save raw data" class="Bool (strict)"("Value"=w1485) -> ()  [unwired: 2 in, 2 out]
        n706 = Enqueue Element(queue=w1484, element=w1480, error in (no error)=w1483) -> ()  [unwired: 1 in, 3 out]
      }
      event "save flag": Value Change {
        n707 = event-data() -> ("NewVal"=w1487:bool)  [unwired: 1 in]
        n708 = To Variant(anything=w1487) -> (Variant=w1491:variant)
        n709 = Bundle(cluster=w1490, "state"=state."dat_update_save_flag", "value"=w1491) -> (w1492:cluster{"state":T8, "value":variant})
        n710 = Enqueue Element(queue=w1489, element=w1492, error in (no error)=w1488) -> ()  [unwired: 1 in, 3 out]
      }
      event "view error anal": Value Change {
        n711 = event-data() -> ("NewVal"=w1494:bool)  [unwired: 1 in]
        n712 = vi-ref "error_anal.vi"() -> (w1493:refnum<vi>)
        n713 = case shown="False" w1494 {
          tunnel: w1493 -> [w1499 w1502]
          tunnel: [w1497 w1501] -> w1495
          tunnel: [w1498 w1500] -> w1496
          frame False {
            n714 = invoke class="VI" method="FP.Close"(reference=w1499) -> (reference out=w1498:refnum<vi>, error out=w1497:errorcluster)  [unwired: 2 in, 1 out]
          }
          frame True {
            n715 = invoke class="VI" method="FP.Open"(reference=w1502) -> (reference out=w1500:refnum<vi>, error out=w1501:errorcluster)  [unwired: 4 in, 3 out]
          }
        }
        n716 = Close Reference(reference=w1496, error in (no error)=w1495) -> ()  [unwired: 1 out]
      }
      event "view full data": Value Change {
        n717 = event-data() -> ("NewVal"=w1506:bool)  [unwired: 1 in]
        n718 = vi-ref "view_full_data.vi"() -> (w1505:refnum<vi>)
        n719 = case shown="True" w1506 {
          tunnel: w1505 -> [w1509 w1512]
          tunnel: [w1507 w1511] -> w1503
          tunnel: [w1508 w1510] -> w1504
          frame False {
            n720 = invoke class="VI" method="FP.Close"(reference=w1509) -> (reference out=w1508:refnum<vi>, error out=w1507:errorcluster)  [unwired: 2 in, 1 out]
          }
          frame True {
            n721 = invoke class="VI" method="FP.Open"(reference=w1512) -> (reference out=w1510:refnum<vi>, error out=w1511:errorcluster)  [unwired: 4 in, 3 out]
          }
        }
        n722 = Close Reference(reference=w1504, error in (no error)=w1503) -> ()  [unwired: 1 out]
      }
      event "ts_plot_lin-log": Value Change {
        n723 = event-data() -> ("NewVal"=w1514:bool)  [unwired: 1 in, 5 out]
        n724 = Boolean To (0,1)(Boolean=w1514) -> (0, 1=w1513:i16)
        n725 = property on="Waveform Graph" class="WFGraph (strict)"("YScale.Mapping Mode"=w1513) -> ()  [unwired: 2 in, 2 out]
      }
      event Key Down {
        n726 = event-data() -> ("Char"=w1516:i16)  [unwired: 1 in, 9 out]
        "Char" <- w1516
        n727 = disable-structure shown="Disabled" {
          disable-tunnel: w1516 -> [w1517 _]
          frame Disabled {
            n728 = case shown="49" w1517 {
              frame 0, Default {
              }
              frame 49 {
                n729 = property on="stage position(s)" class="Arr (strict)"("Array Element.Key Focus"=TRUE) -> ()  [unwired: 2 in, 2 out]
              }
              frame 98 {
                n730 = property on="get bg" class="Bool (strict)"() -> ("Value"=w1520:bool)  [unwired: 2 in, 2 out]
                n731 = Not(x=w1520) -> (.not. x?=w1519:bool)
                n732 = property on="get bg" class="Bool (strict)"("Val(Sgnl)"=w1519) -> ()  [unwired: 2 in, 2 out]
              }
              frame 99 {
                n733 = property on="cont acq" class="Bool (strict)"() -> ("Value"=w1522:bool)  [unwired: 2 in, 2 out]
                n734 = Not(x=w1522) -> (.not. x?=w1521:bool)
                n735 = property on="cont acq" class="Bool (strict)"("Val(Sgnl)"=w1521) -> ()  [unwired: 2 in, 2 out]
              }
              frame 115 {
                n736 = property on="get_single_acq" class="Bool (strict)"("Val(Sgnl)"=TRUE ("Value (Signaling)")) -> ()  [unwired: 2 in, 2 out]
              }
            }
          }
          frame Enabled {
          }
        }
        n737 = Wait (ms)(milliseconds to wait=u32 75) -> ()  [unwired: 1 out]
      }
      event Panel Close? {
        w1529 = TRUE
        n738 = event-data() -> ()  [unwired: 1 in, 4 out]
        n739 = Bundle(cluster=w1526, "state"=state."stop" ("element")) -> (w1524:cluster{"state":T8, "value":variant})  [unwired: 1 in]
        n740 = Enqueue Element(queue=w1528, element=w1524, error in (no error)=w1527) -> ()  [unwired: 1 in, 3 out]
        n741 = event-data("Discard?"=w1529) -> ()  [unwired: 1 in, 1 out]
      }
    }
  }
  n742 = call <vilib>:"Simple Error Handler.vi"("error in (no error)"=w128) -> ()  [unwired: 4 in, 5 out]
